vi "IV_Sweep_tool_Probe_Station_Resistance_measure_16_0202.vi"() -> ()   [LabVIEW 2013]
doc: "I. Description:\nThis example demonstrates how to continuously acquire and generate data at the same time, synchronized with one another.\n\nII. Instructions for Running:\n1. Select the physical channel to correspond to where your signal is input on the DAQ device. Also, select the corresponding channel for where your signal is being generated.\n2. Enter the minimum and maximum voltage ranges.\nNote: For better accuracy try to match the input range to the expected voltage level of the measured signal.\n3. Set the sample rate of the acquisition.\nNote: The rate should be at least twice as fast as the maximum frequency component of the signal being acquired. \n6. Select the Rate for the generation\n7. Select what type of signal to generate and the amplitude.\nNote: This example requires two DMA channels to run. If your hardware does not support two DMA channels, you need to set the Data Transfer Mechanism property for the Analog Output Task to use \"Interrupts\". The Data Transfer Mechanism property is located in the DAQmx Channel Property hierarchy at:\n\nDAQmx Channel Property Node>>Analog Output>>General Properties>>Advanced>>Data Transfer and Memory>>Data Transfer Mechanism\n\nRefer to your device documentation to determine how many DMA channels are supported for your hardware.\n\nIII. Block Diagram Steps:\n1. Create an analog input voltage channel. Also, create an analog output voltage channel.\n2. Set the rate for the sample clock. Additionally, define the sample mode to be continuous. Also, set the sample clock rate for the signal generation.\n2a. Call the Get Terminal Name with Device Prefix VI. This will take a Task and a terminal and create a properly formatted device + terminal name to use as the source of the Trigger.\n3. Define the parameters for a Digital Edge Start Trigger. Set the Analog output to trigger off the AI Start Trigger. This is an internal trigger signal.\n4. Use the Basic Function Generator VI to create the signal to be generated.\n5. Call the Start VI to arm the two functions. Make sure the analog output is armed before the analog input. This will ensure both will start at the same time.\n6. Read the waveform data in a loop until the user hits the stop button or an error occurs. The Is Task Done? VI is used to check for errors in the Analog Output Task.\n7. Call the Clear VI to Clear the Task\n8. Use the popup dialog box to display an error if any.\n\nIV. I/O Connections Overview:\nMake sure your signal input/output terminals match the Physical Channel I/O controls."
uses:
  <vilib>/Utility/error.llb/DialogType.ctl
  <vilib>/DAQmx/write.llb/DAQmx Write (Analog 2D DBL NChan NSamp).vi
  <vilib>/DAQmx/read.llb/DAQmx Read (Analog 1D DBL NChan 1Samp).vi
  <vilib>/DAQmx/write.llb/DAQmx Write (Analog DBL 1Chan 1Samp).vi
  <vilib>/DAQmx/read.llb/DAQmx Read (Analog DBL 1Chan 1Samp).vi
  <vilib>/Analysis/baseanly.llb/Mean (DBL).vi
  <vilib>/DAQmx/write.llb/DAQmx Write (Analog 1D DBL NChan 1Samp).vi
  <vilib>/DAQmx/create/channels.llb/DAQmx Create Channel (AO-Voltage-Basic).vi
  <vilib>/DAQmx/create/channels.llb/DAQmx Create Channel (AI-Voltage-Basic).vi
  <vilib>/DAQmx/configure/timing.llb/DAQmx Timing (Sample Clock).vi
  <vilib>/DAQmx/configure/trigger.llb/DAQmx Start Trigger (Digital Edge).vi
  <vilib>/DAQmx/miscellaneous.llb/DAQmx Fill In Error Info.vi
  <vilib>/Utility/file.llb/Write To Spreadsheet File (DBL).vi
  <vilib>/Utility/file.llb/Write To Spreadsheet File (string).vi
  pid/pid.llb/PID (DBL).vi
  pid/pid.llb/PID Output Rate Limiter (DBL).vi
  <vilib>/ptbypt/NI_PtbyPt.lvlib
  <resource>/objmgr/daqmx.rc
  <vilib>/Analysis/NI_AALBase.lvlib
  <vilib>/Analysis/NI_AALPro.lvlib
panel:
  in  "amplif":dbl=-0.01
  out "date/time string":string
  out "Bias Sweep 2":dbl[](graph)
  out "Array":dbl[](array[numeric])
  out "intercept":dbl
  out "Resistance":dbl
  out "RTD-IV":cluster{dbl[], dbl[]}(graph)
  in  "Bias Offset Correct":dbl
  out "Bias Sweep":dbl[](graph)
  out "element":dbl
  out "mean":dbl format="%.6f"
  out "size(s)":i32
  out "Numeric":i32
  in  "PID":bool=TRUE caption="Step Z"
  in  "Tab Control":enum32{"PID Controller", "Tapping Controls"}(tab)=enum."Tapping Controls"
  in  "Proportional Gain":dbl=0.0001
  in  "Integral Gain":dbl=1e-07
  in  "Differential Gain":dbl=1e-05
  in  "Setpoint":dbl=0.1
  in  "Piezo Delta rate":dbl=1000.0
  in  "Min Current":dbl=0.002
  in  "Max Current":dbl=10.2
  in  "Ramp Rate":dbl=20.0
  in  "Make Contact":i32=1200
  in  "Break Contact":i32=500
  in  "Step Length":i32=100
  in  "Step Max":dbl=0.3
  in  "Step Min":dbl=0.05
  out "Tapping Stop":bool
  out "Case":i32
  in  "Contact Cycles":i32
  in  "Tapping":bool caption="Step Z"
  out "x/y":dbl
  out "Waveform Chart":dbl(graph)
  in  "Analog Ouyput 1":dbl(slide) min=-10.0 max=10.0 step=0.001 scale=-10.0..10.0
  in  "Manual Z":bool caption="Step Z"
  in  "Sweep Amplitude":dbl=1.0
  in  "Stop Sweep":bool
  out "Connections 2":string="AI0=Current\nAI1=Bias\nAI2=dI/dV\nAI3=d2I/dV2\nAI4=X-Axis\nAI5=Z-Axis\n"
  out "Connections":string="AO0=Bias\nAO1=Z-axis\nAO2=X-Axis\nAO3=NA"
  out "Save Indicator":bool
  in  "Z-Direction":bool caption="Step Z"
  in  "Update Bias":bool
  in  "Save IV":bool
  in  "Save Decay":bool
  in  "Sweep Bias":bool
  in  "Step Z":bool
  in  "Comment":string="Molecule=TP4\nGain=10nA\nBias Gain=div/1\nSweep Freq.=0.0008Hz\nRef. Bias=4mV\nRef. Freq=2.977kHz\nGain LIA1=2mV\nTC LIA1=1s\nGain LIA2=5mV\nTC LIA2=1s\nLIA1=EGG\nLIA2=SRS\nEGG is driving(possible 5mV offset)"
  in  "Filenumber":i32
  in  "DATA Filename":string="Data_"
  in  "Data Directory":path=path "E:/Research/Data"
  out "Current Decay":cluster{dbl[], dbl[]}(graph)
  out "d2I/dV2":cluster{dbl[], dbl[]}(graph)
  out "dI/dV":cluster{dbl[], dbl[]}(graph)
  out "IV":cluster{dbl[], dbl[]}(graph)
  in  "# Samples":i32=2000
  in  "Frequency (Hz)":dbl=1.0
  out "Measurement 2":cluster{i32, dbl, dbl[]}(graph) caption="Measurement"
  out "Actual Update Generation Rate 2":dbl=5000.0 caption="Actual Update Generation Rate" format="%0.2f"
  in  "stop 3":bool
  in  "Bias":dbl=0.1 caption="Bias Start Point" step=0.1 format="%_3g"
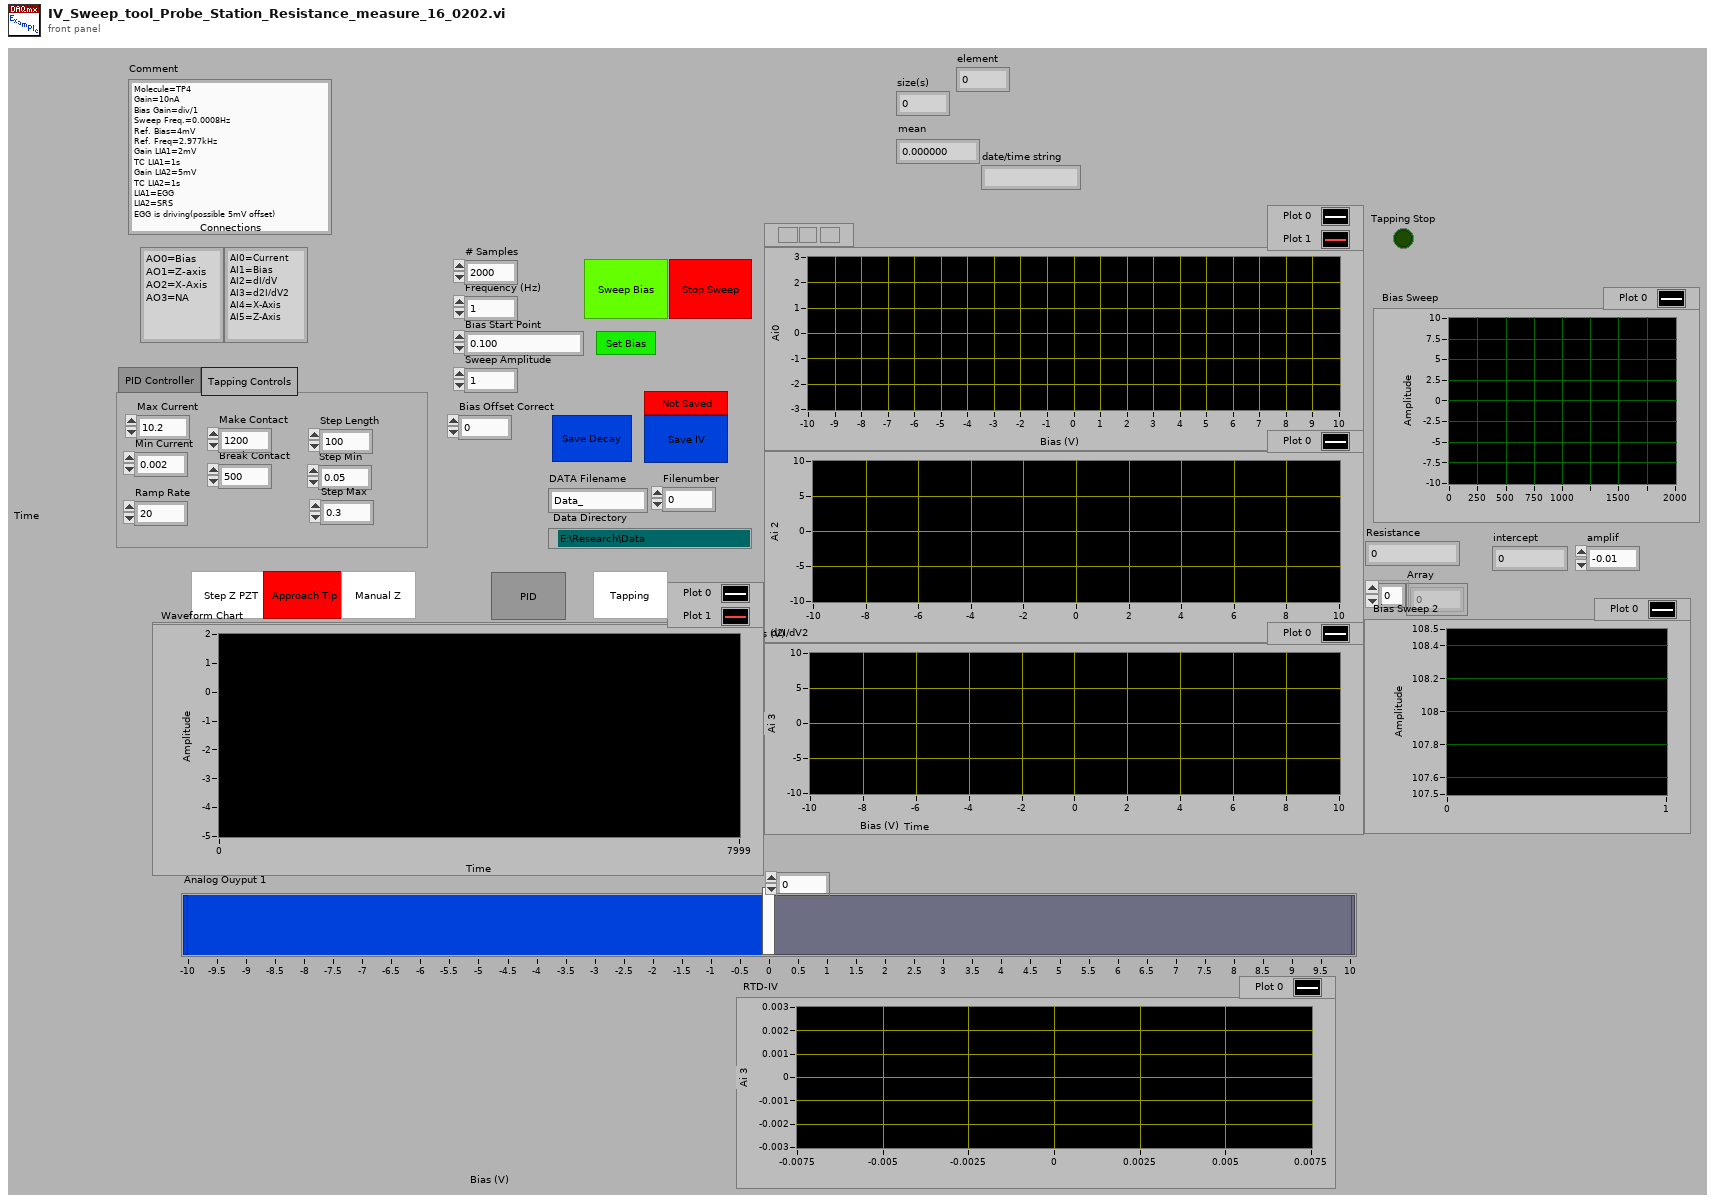
[diagram p1: front panel]
types:
  T1 = enum16{"open", "replace", "create", "open or create", "replace or create", "replace or create with confirmation"}
  T2 = typedef "DialogType.ctl" = u16
  T3 = cluster{"Proportional Gain":dbl, "Integral Gain ":dbl, "Differential Gain":dbl}
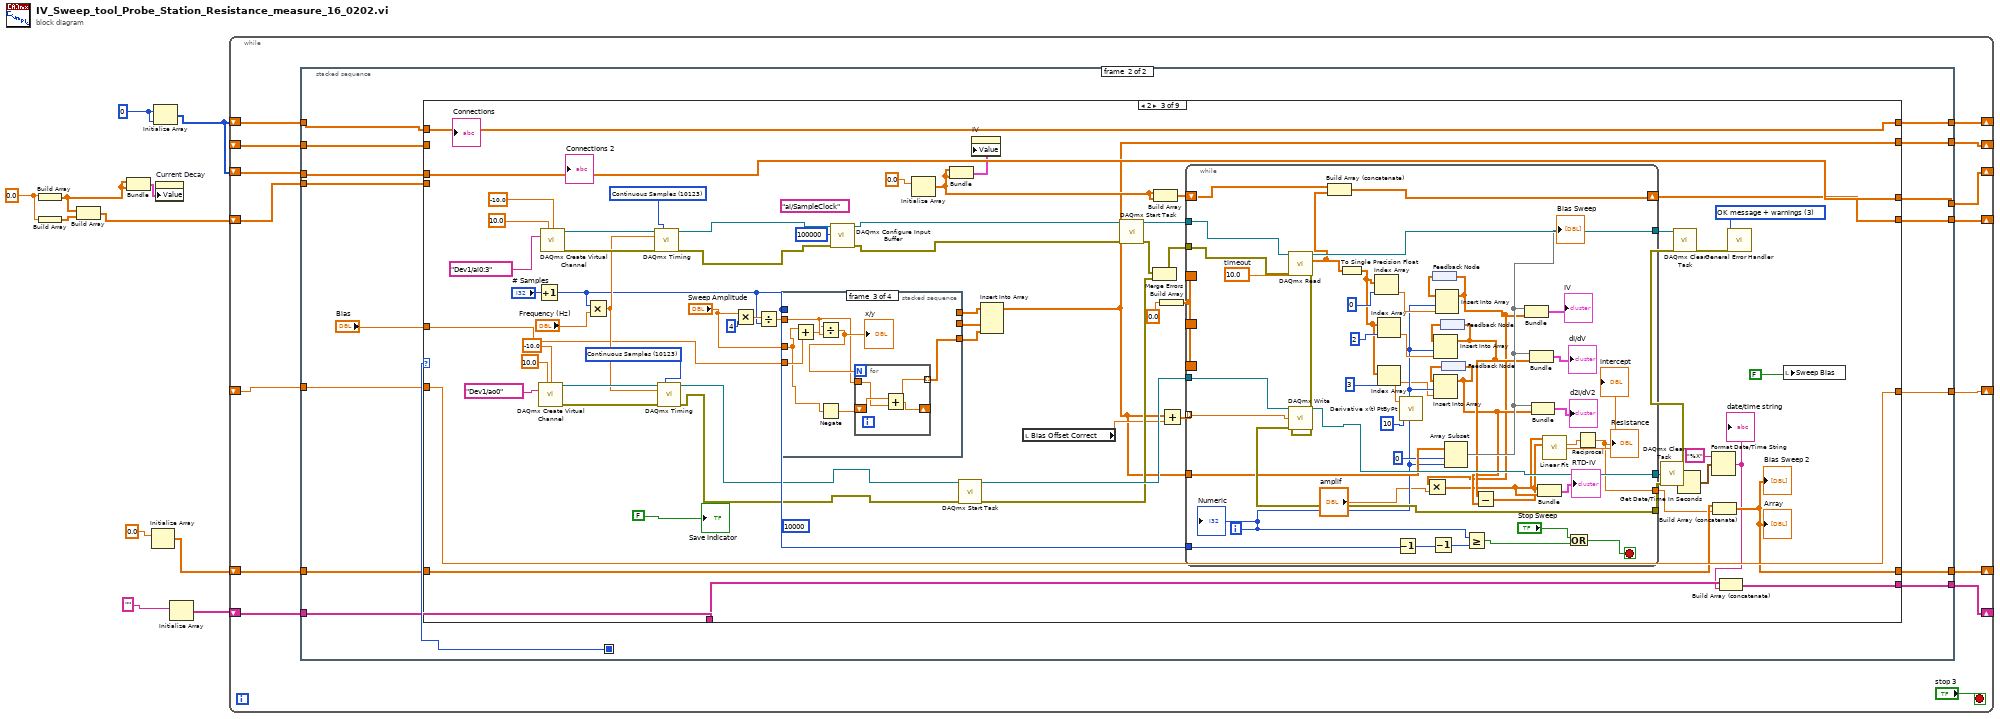
[diagram p0: block diagram]
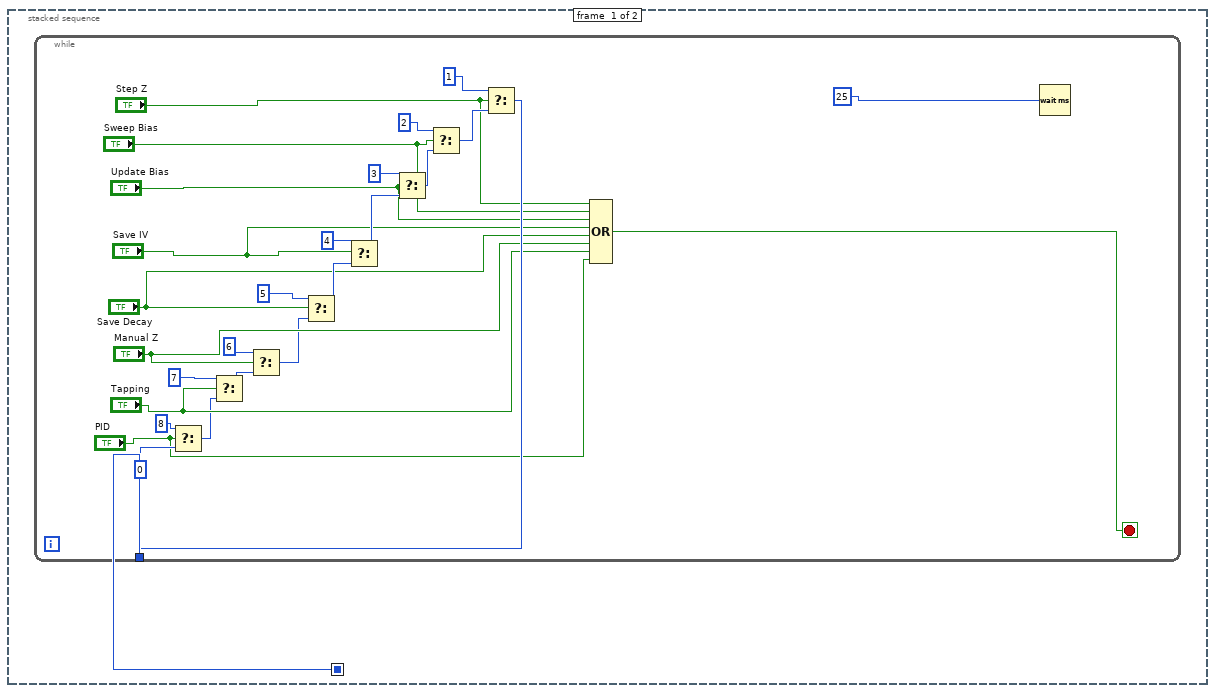
[diagram p2: hidden frame]
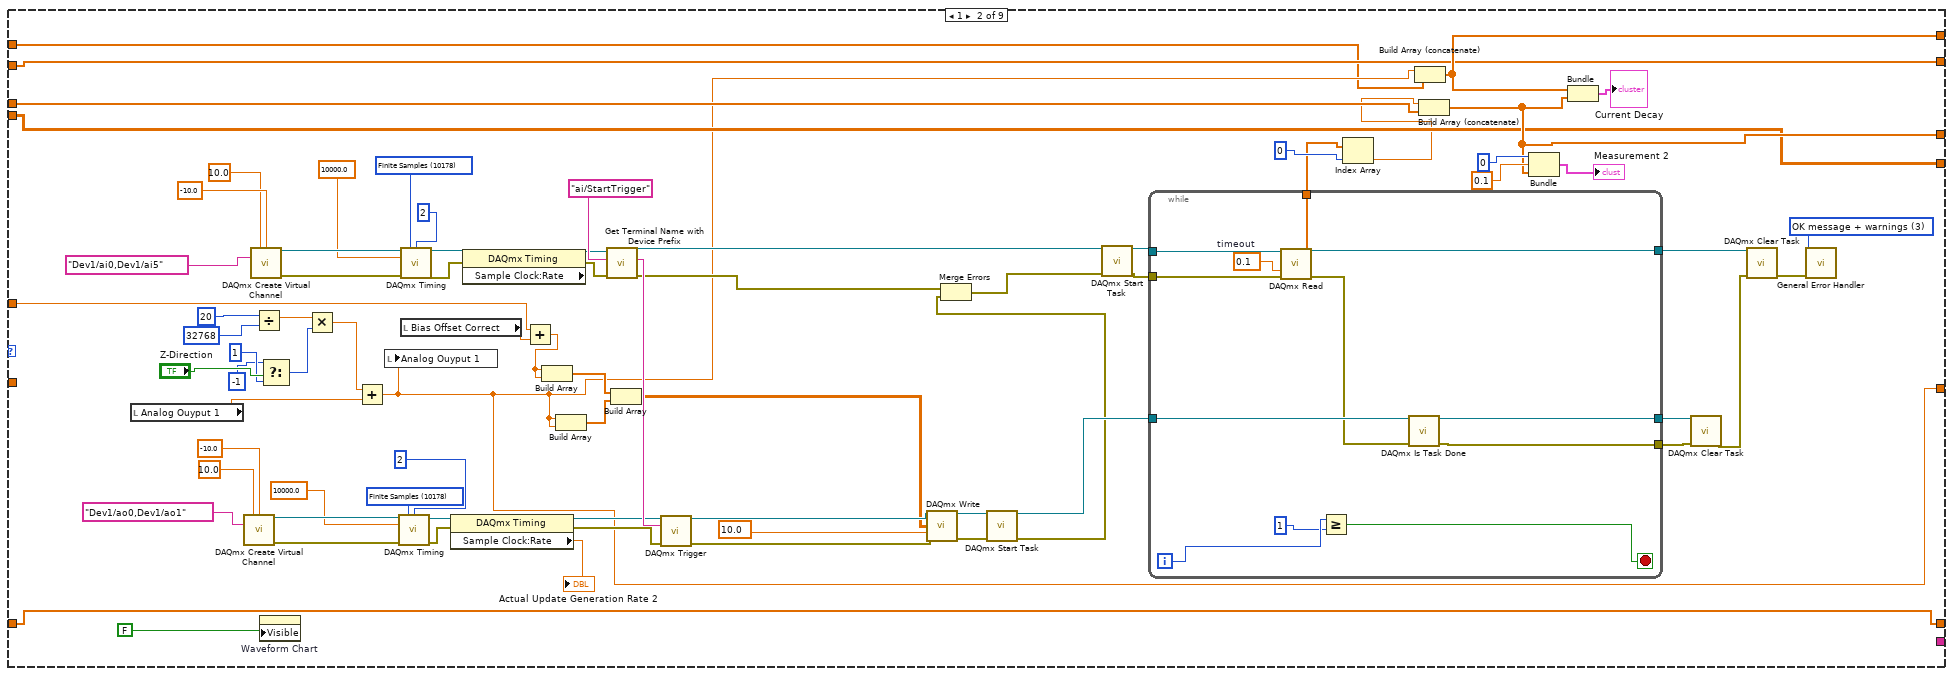
[diagram p4: hidden frame]
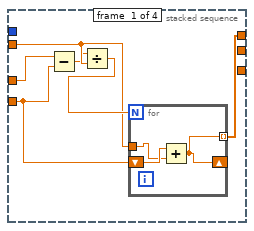
[diagram p5: hidden frame]
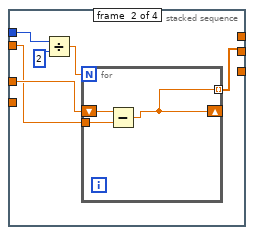
[diagram p6: hidden frame]
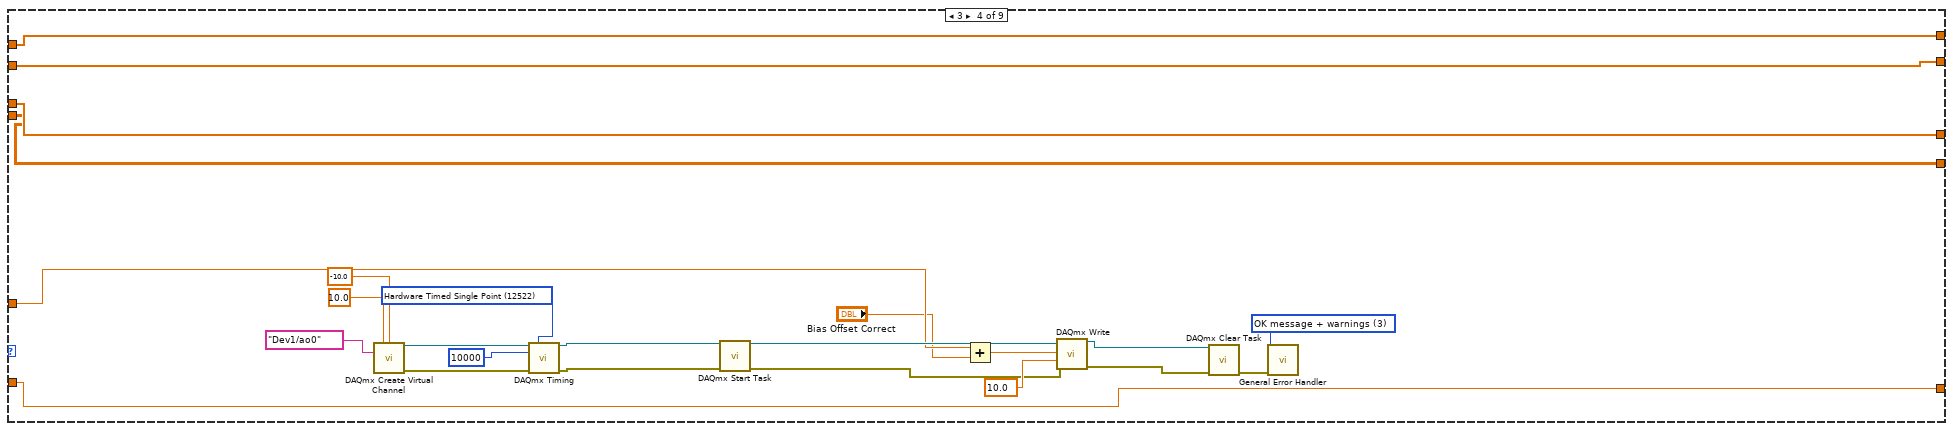
[diagram p8: hidden frame]
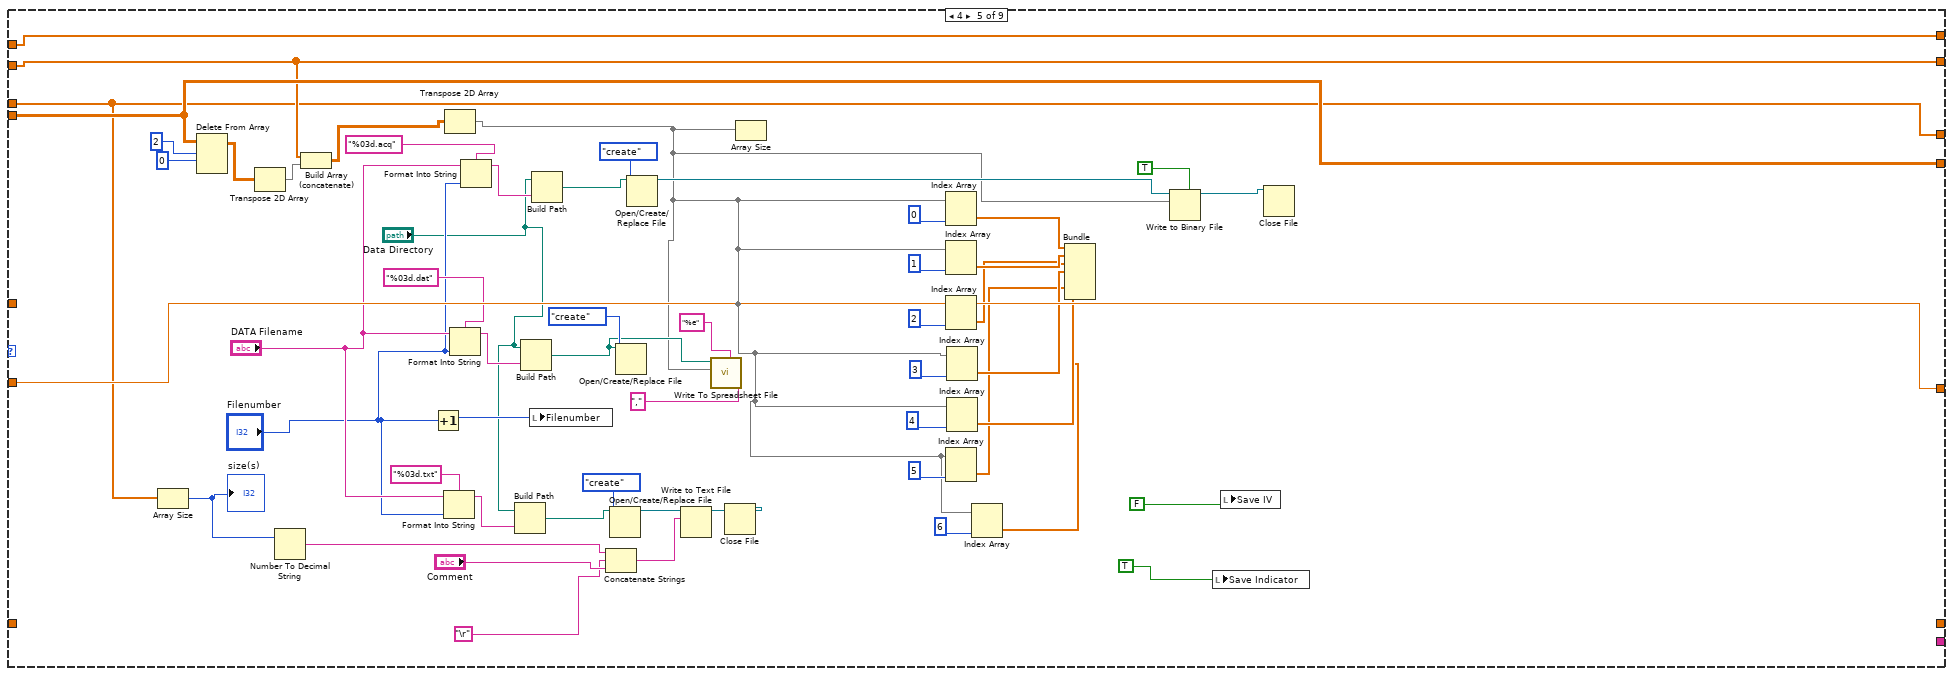
[diagram p9: hidden frame]
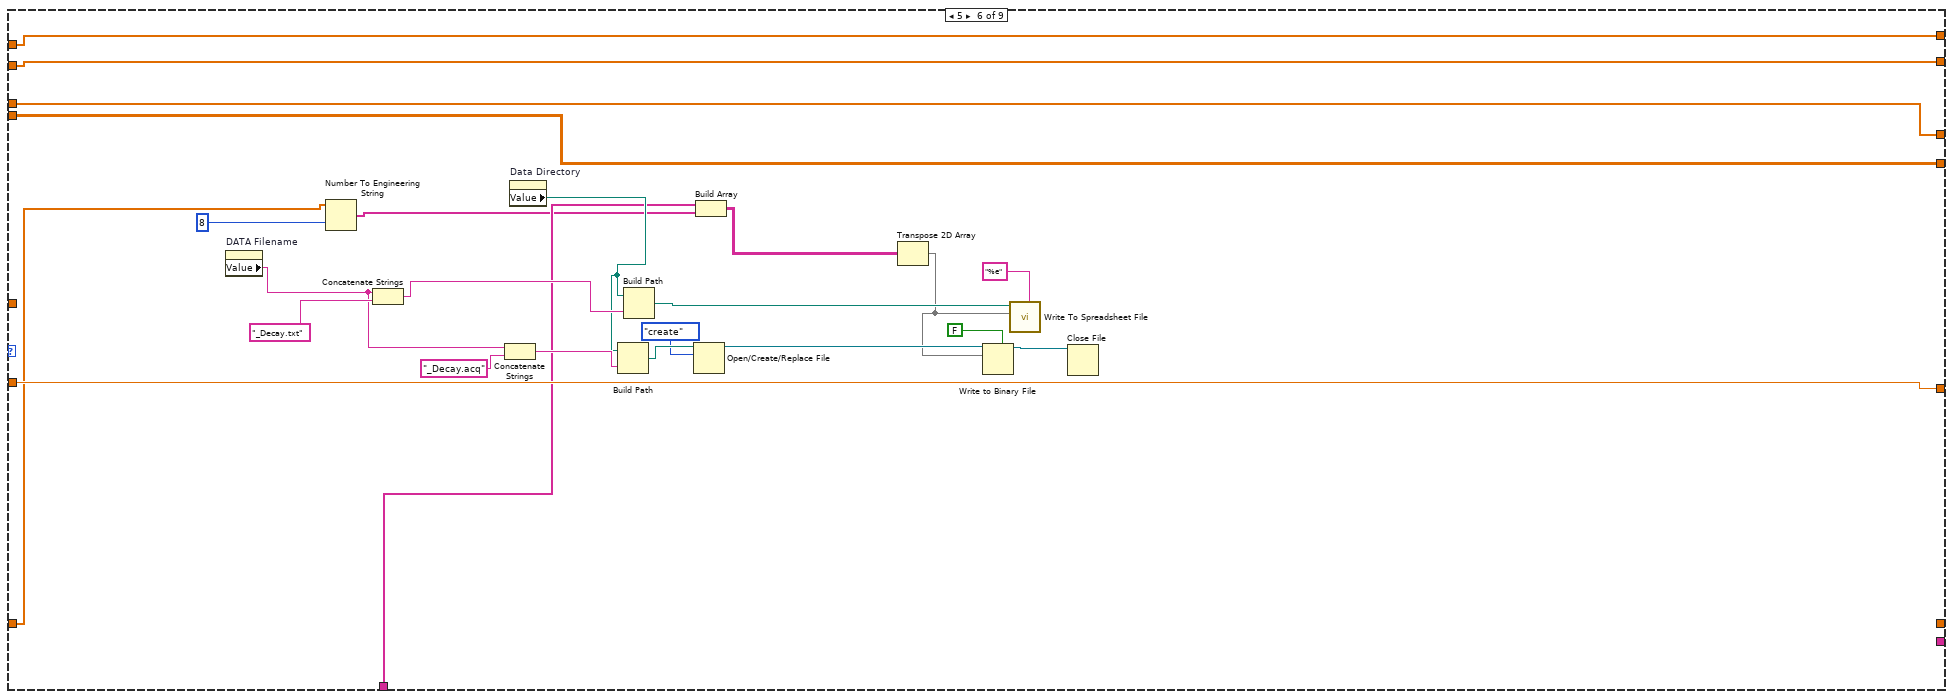
[diagram p10: hidden frame]
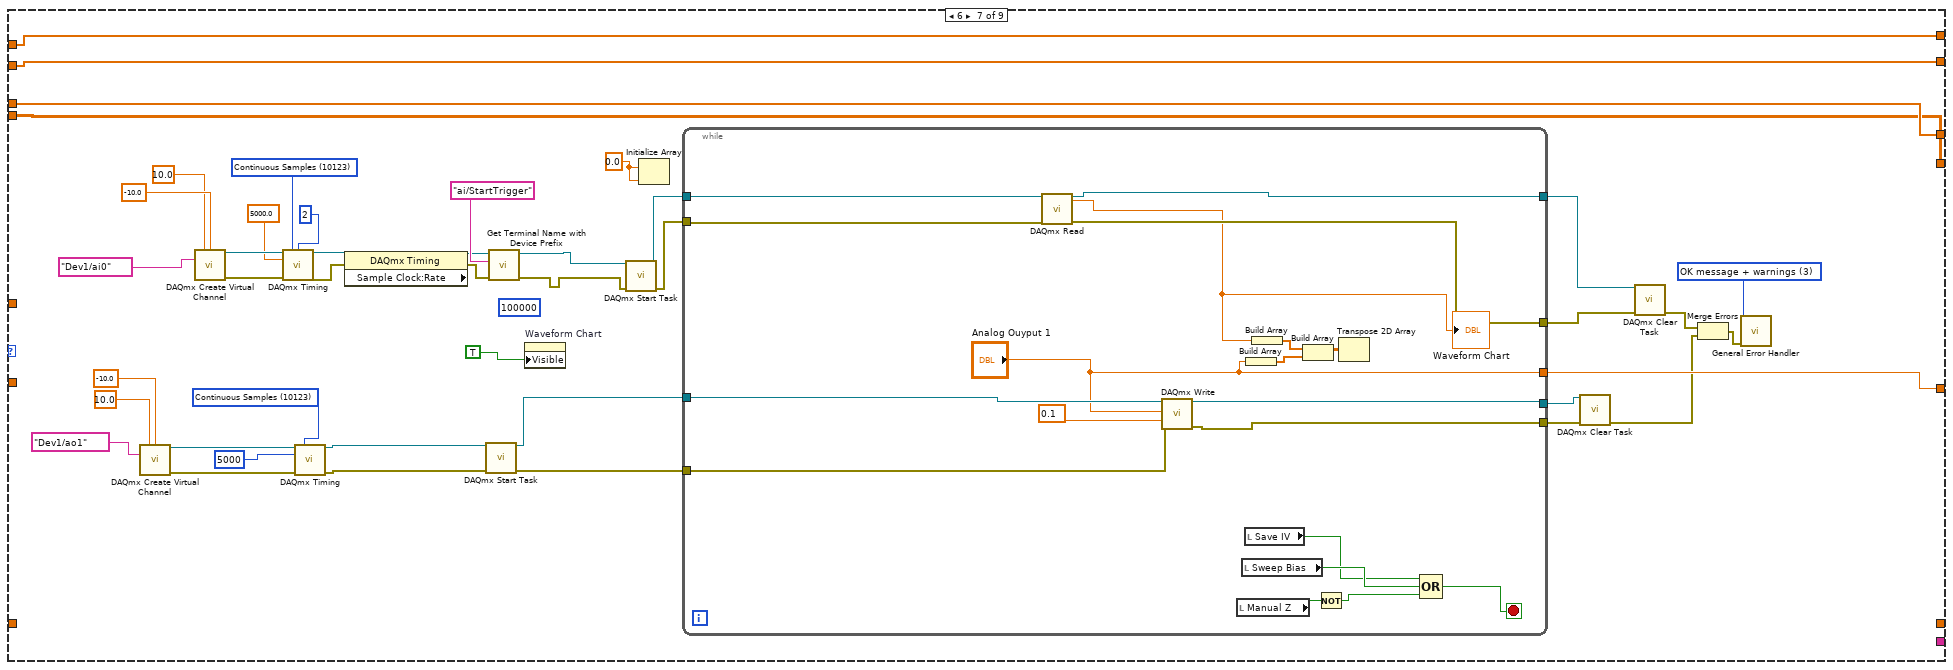
[diagram p11: hidden frame]
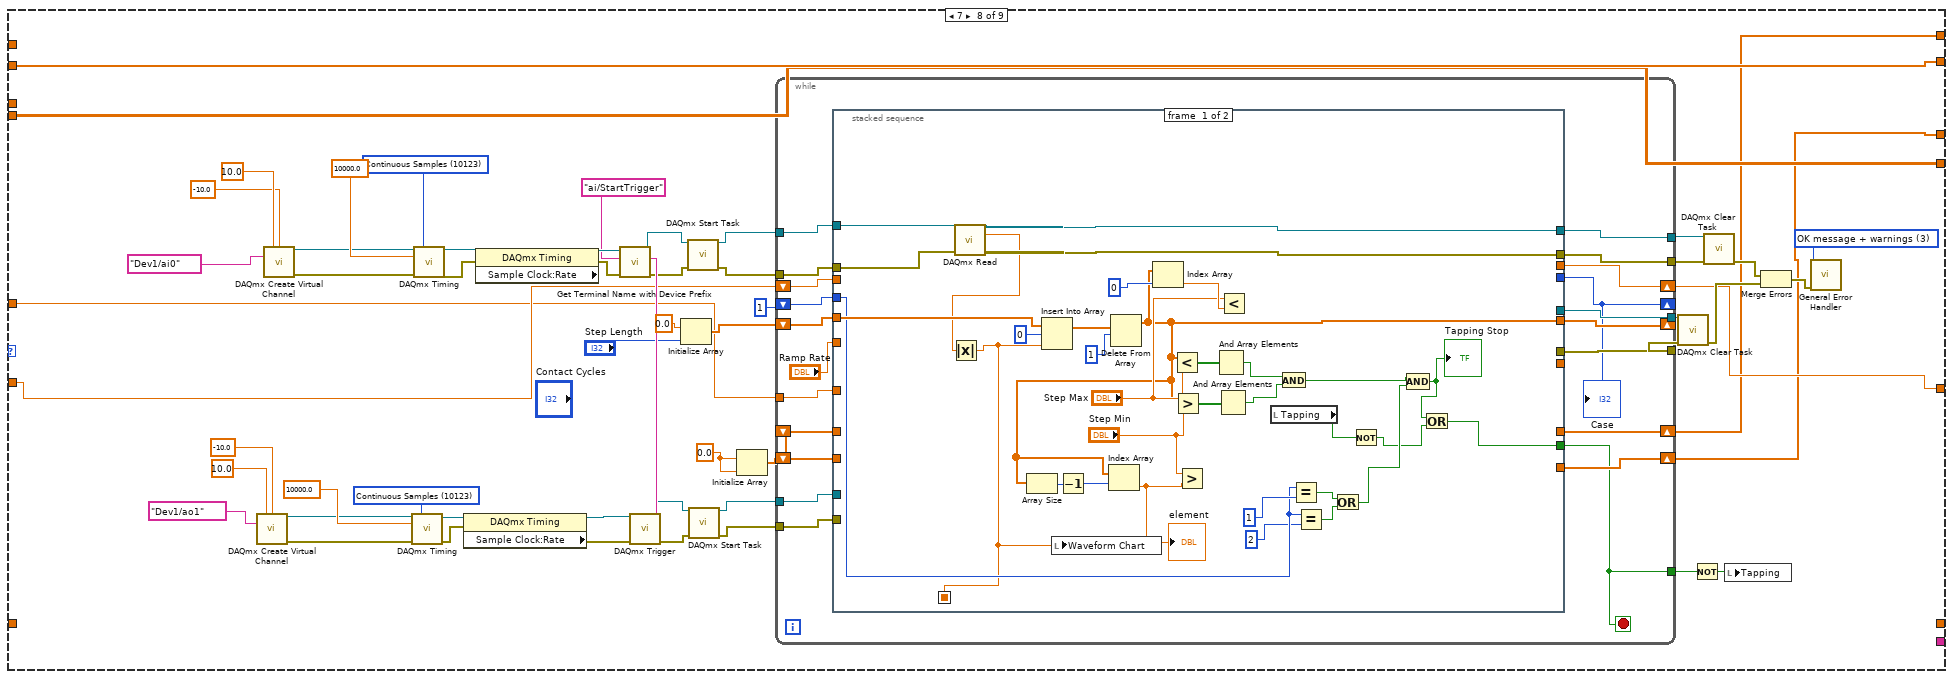
[diagram p12: hidden frame]
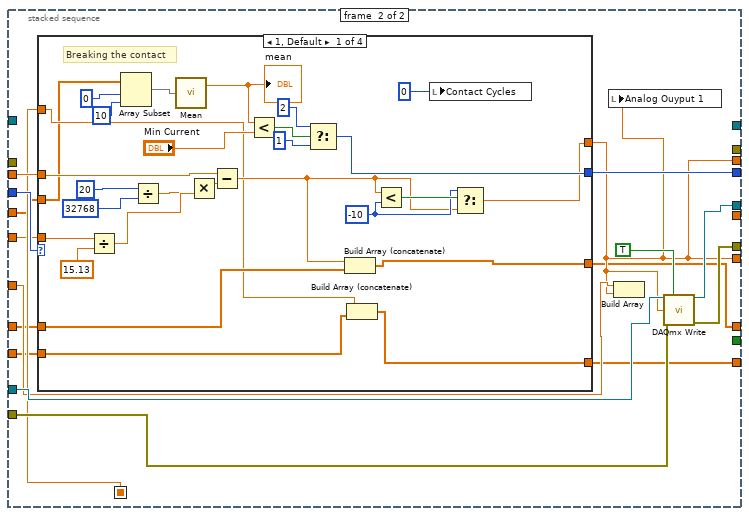
[diagram p13: hidden frame]
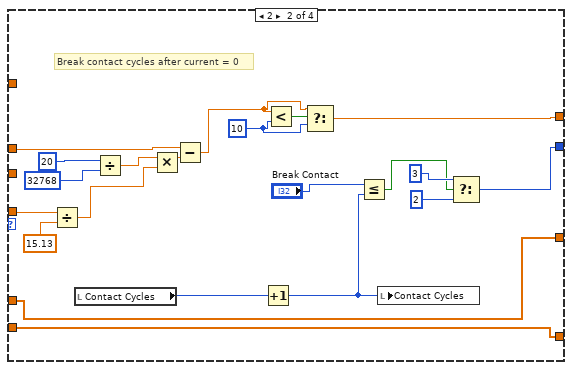
[diagram p14: hidden frame]
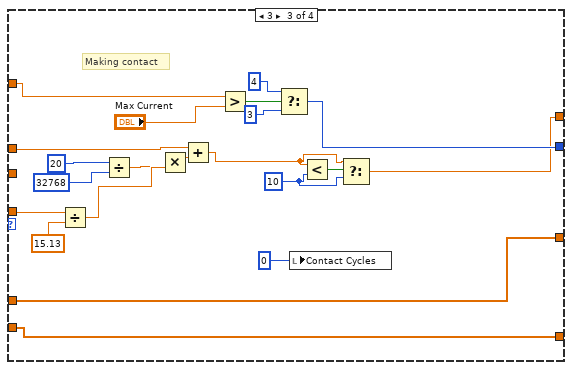
[diagram p15: hidden frame]
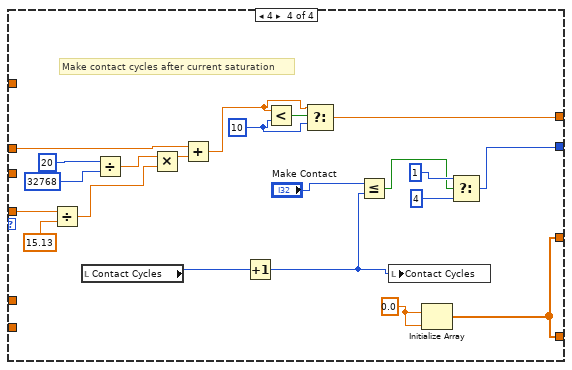
[diagram p16: hidden frame]
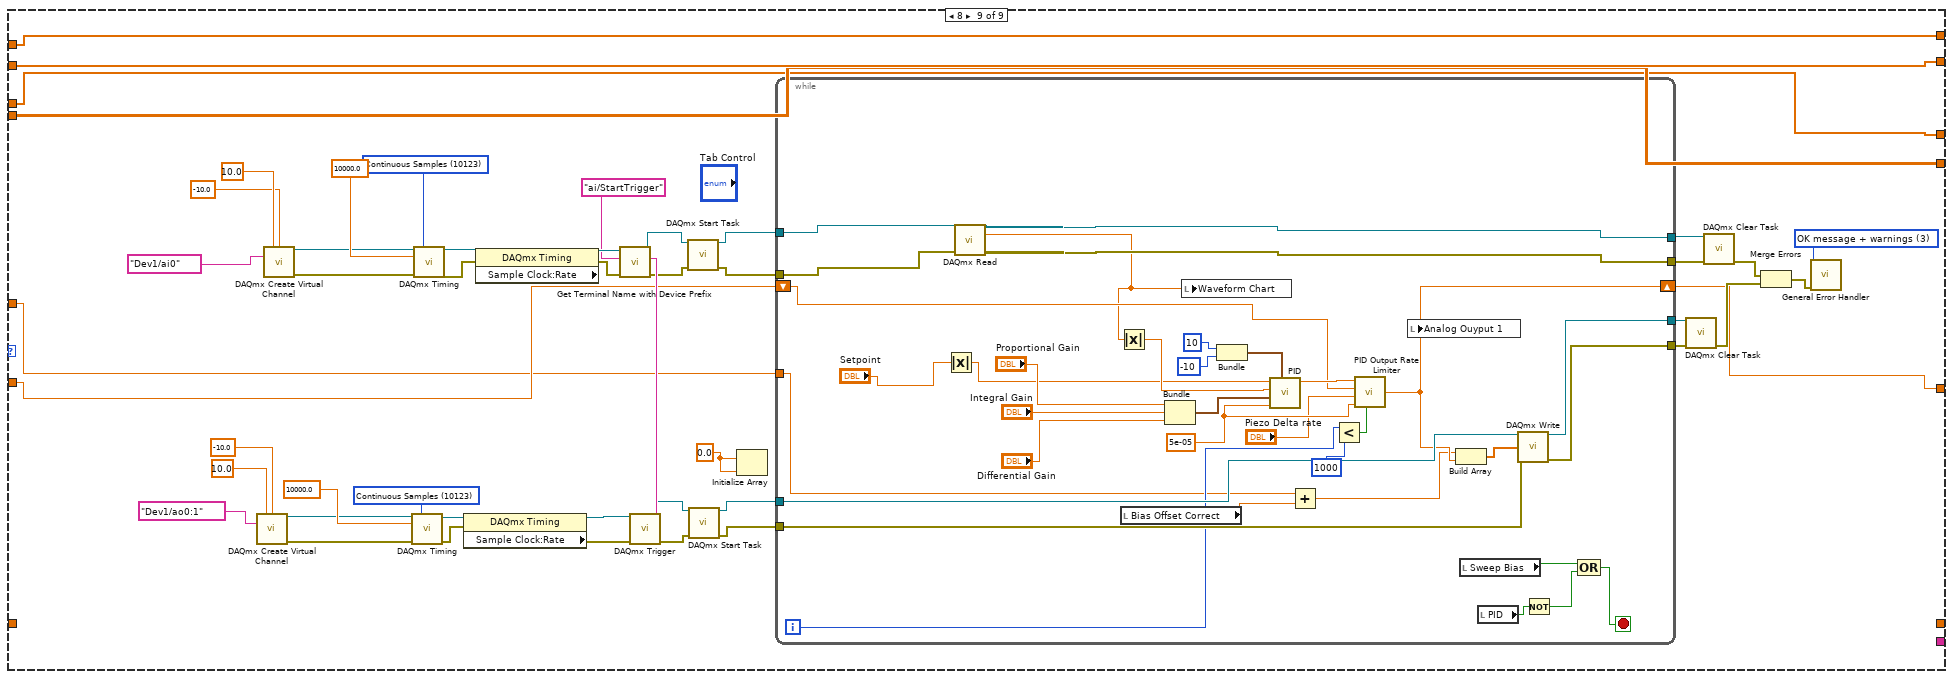
[diagram p17: hidden frame]
diagram:
  w6 = 0
  w11 = 0.0
  n1 = Build Array(w11) -> (w8:dbl[])
  n2 = Build Array(w11) -> (w10:dbl[])
  n3 = Build Array(w8, w10) -> (w9:dbl[][])
  n4 = Bundle(w8, w8) -> (w7:cluster{dbl[], dbl[]})  [unwired: 1 in]
  n5 = Initialize Array(0.0) -> (w3:dbl[])  [unwired: 1 in]
  n6 = Initialize Array(w6, w6) -> (w5:i32[])
  n7 = property on="Current Decay" class="XYGraph (strict)"("Value"=w7) -> ()  [unwired: 2 in, 2 out]
  n8 = Initialize Array("") -> (w1:string[])  [unwired: 1 in]
  n9 = while {
    shift-right: [w24] -> _
    shift-left: w5 -> [w25]
    shift-right: [w22] -> _
    shift-left: w5 -> [w23]
    shift-right: [w20] -> _
    shift-left: _ -> [w21]
    shift-right: [w18] -> _
    shift-left: w9 -> [w19]
    shift-right: [w16] -> _
    shift-left: _ -> [w17]
    shift-right: [w15] -> _
    shift-left: w3 -> [w14]
    shift-right: [w12] -> _
    shift-left: w1 -> [w13]
    stop <- "stop 3" stop-if-true
    n10 = stacked-sequence {
      seq-local: [w27 _] -> [_ w70]
      tunnel: w25 -> [_ w69]
      tunnel: [_ w68] -> w24
      tunnel: w23 -> [_ w66]
      tunnel: [_ w65] -> w22
      tunnel: w21 -> [_ w64]
      tunnel: [_ w59] -> w20
      tunnel: w19 -> [_ w63]
      tunnel: [_ w62] -> w18
      tunnel: w17 -> [_ w61]
      tunnel: [_ w60] -> w16
      tunnel: w14 -> [_ w58]
      tunnel: [_ w57] -> w15
      tunnel: w13 -> [_ w56]
      tunnel: [_ w55] -> w12
      frame #0 {
        n11 = while {
          tunnel: [w45] -> w27
          stop <- w44 stop-if-true
          n12 = Select(t=8, s="PID", f=0) -> (s? t:f=w31:i32)
          n13 = Select(t=7, s="Tapping", f=w31) -> (s? t:f=w33:i32)
          n14 = Select(t=6, s="Manual Z", f=w33) -> (s? t:f=w34:i32)
          n15 = Select(t=5, s="Save Decay", f=w34) -> (s? t:f=w50:i32)
          n16 = Select(t=4, s="Save IV", f=w50) -> (s? t:f=w49:i32)
          n17 = Select(t=3, s="Update Bias", f=w49) -> (s? t:f=w47:i32)
          n18 = Select(t=2, s="Sweep Bias", f=w47) -> (s? t:f=w54:i32)
          n19 = Select(t=1, s="Step Z", f=w54) -> (s? t:f=w45:i32)
          n20 = Compound Arithmetic op=OR("Step Z", "Sweep Bias", "Update Bias", "Save IV", "Save Decay", "Manual Z", "Tapping", "PID") -> (w44:bool)
          n21 = Wait (ms)(milliseconds to wait=25) -> ()  [unwired: 1 out]
        }
      }
      frame #1 {
        n22 = case shown="2" w70 {
          tunnel: w69 -> [w77 w85 w214 w312 w332 w388 w448 _ w688]
          tunnel: [w77 w98 w214 w312 w332 w388 w448 w474 w688] -> w68
          tunnel: "Bias" -> [_ w81 w199 w306 _ _ _ w480 w687]
          tunnel: w66 -> [w76 w82 w211 w313 w379 w404 w450 _ w689]
          tunnel: [w76 w99 w211 w313 w379 w404 w450 w475 w689] -> w65
          tunnel: w64 -> [w75 _ w210 w311 w378 w405 _ w481 w696]
          tunnel: [w75 w83 w210 w311 w378 w405 w419 w476 w693] -> w59
          tunnel: w63 -> [w74 w96 _ w309 w358 w406 w447 w478 w694]
          tunnel: [w74 w96 w191 w309 w358 w406 w447 w478 w694] -> w62
          tunnel: [w73 w91 w174 w308 w356 w389 w449 w479 w695] -> w60
          tunnel: w61 -> [w73 w91 _ w308 w356 w389 w449 w479 w695]
          tunnel: w58 -> [w72 w78 w173 _ _ w386 _ _ _]
          tunnel: [w72 w78 w171 _ _ _ _ _ _] -> w57
          tunnel: w56 -> [w71 _ w170 _ _ w387 _ _ _]
          tunnel: [w71 _ w169 _ _ _ _ _ _] -> w55
          frame 0, Default {
          }
          frame 1 {
            w133 = T2 3 items=["no dialog", "OK message", "continue or stop message", "OK message + warnings", "continue/stop + warnings"] ("type of dialog (OK msg:1)")
            w145 = 10178 items=["Finite Samples"=10178, "Continuous Samples"=10123] ("sample mode")
            w150 = 10178 items=["Finite Samples"=10178, "Continuous Samples"=10123] ("sample mode")
            n23 = local read "Analog Ouyput 1"() -> (w86:dbl)
            n24 = call-poly <vilib>:"DAQmx Create Virtual Channel.vi"("maximum value"=10.0 ("maximum value 2"), "minimum value"=-10.0 ("minimum value 2"), "physical channels"=tag "Dev1/ao0,Dev1/ao1" ("physical channels 2")) -> ("task out"=w144:refnum<k21>, "error out"=w143:errorcluster)  [unwired: 11 in]
            n25 = call-poly <vilib>:"DAQmx Create Virtual Channel.vi"("maximum value"=10.0 ("Maximum Value 2"), "minimum value"=-10.0 ("Minimum Value 2"), "physical channels"=tag "Dev1/ai0,Dev1/ai5" ("Physical Channel 2")) -> ("task out"=w148:refnum<k21>, "error out"=w149:errorcluster)  [unwired: 11 in]
            n26 = Divide(x=20, y=32768) -> (x/y=w95:dbl)
            n27 = property on="Waveform Chart" class="WFChart (strict)"("Visible"=FALSE) -> ()  [unwired: 2 in, 2 out]
            n28 = Select(t=-1 ("f"), s="Z-Direction", f=1) -> (s? t:f=w93:i32)
            n29 = Multiply(x=w95, y=w93) -> (x*y=w94:dbl)
            n30 = Add(x=w94, y=w86) -> (x+y=w83:dbl)
            n31 = local write "Analog Ouyput 1"(w83) -> ()
            n32 = call-poly <vilib>:"DAQmx Timing.vi"("task/channels in"=w144, "sample mode"=w145, "samples per channel"=2, "rate"=10000.0 ("rate 2"), "error in"=w143) -> ("task out"=w128:refnum<k21>, "error out"=w127:errorcluster)  [unwired: 9 in]
            n33 = call-poly <vilib>:"DAQmx Timing.vi"("task/channels in"=w148, "sample mode"=w150, "samples per channel"=2, "rate"=10000.0 ("Rate 2"), "error in"=w149) -> ("task out"=w122:refnum<k21>, "error out"=w121:errorcluster)  [unwired: 9 in]
            n34 = local read "Bias Offset Correct"() -> (w80:dbl)
            n35 = property class="DAQmx Timing"(reference=w128, error in=w127) -> (reference out=w129:refnum<k21>, error out=w126:errorcluster, "Sample Clock:Rate"=→"Actual Update Generation Rate 2":dbl)
            n36 = property class="DAQmx Timing" props=["Sample Clock:Rate"](reference=w122, error in=w121) -> (reference out=w120:refnum<k21>, error out=w119:errorcluster)  [unwired: 1 out]
            n37 = Add(x=w81, y=w80) -> (x+y=w79:dbl)
            n38 = Build Array(w79, w79) -> (w106:dbl[])
            n39 = Build Array(w83, w83) -> (w105:dbl[])
            n40 = call "Get Terminal Name with Device Prefix.vi"("error in (no error)"=w119, "Local Terminal Name"="ai/StartTrigger" ("terminal"), "task/channels in"=w120) -> ("error out"=w125:errorcluster, "Terminal Name with Device Prefix"=w130:tag, "task out"=w110:refnum<k21>)  [unwired: 6 in]
            n41 = Build Array(w106, w105) -> (w104:dbl[][])
            n42 = call-poly <vilib>:"DAQmx Trigger.vi"("task/channels in"=w129, "source"=w130, "error in"=w126) -> ("task out"=w135:refnum<k21>, "error out"=w136:errorcluster)  [unwired: 11 in]
            n43 = call-poly <vilib>:"DAQmx Write.vi"("task/channels in"=w135, "data"=w104, "timeout"=10.0 ("Wirite Timeout"), "error in"=w136) -> ("task out"=w138:refnum<k21>, "error out"=w137:errorcluster)  [unwired: 9 in, 1 out]
            n44 = call <vilib>:"DAQmx Start Task.vi"("task/channels in"=w138, "error in"=w137) -> ("task out"=w142:refnum<k21>, "error out"=w124:errorcluster)  [unwired: 12 in]
            n45 = Merge Errors(w125, w124) -> (w112:errorcluster)
            n46 = call <vilib>:"DAQmx Start Task.vi"("task/channels in"=w110, "error in"=w112) -> ("task out"=w109:refnum<k21>, "error out"=w111:errorcluster)  [unwired: 12 in]
            n47 = while {
              tunnel: [w165] -> w151
              tunnel: w142 -> [w164]
              tunnel: [w163] -> w141
              tunnel: w109 -> [w154]
              tunnel: [w162] -> w118
              tunnel: [w159] -> w102
              tunnel: w111 -> [w155]
              i -> [w158]
              stop <- w156 stop-if-true
              w161 = 0.1  # timeout
              n48 = call-poly <vilib>:"DAQmx Read.vi"("task/channels in"=w154, "timeout"=w161, "error in"=w155) -> ("task out"=w165:refnum<k21>, "data"=w159:dbl[], "error out"=w160:errorcluster)  [unwired: 10 in]
              n49 = Greater Or Equal?(x=w158, y=1) -> (x >= y?=w156:bool)
              n50 = call <vilib>:"DAQmx Is Task Done.vi"("task/channels in"=w164, "error in"=w160) -> ("task out"=w163:refnum<k21>, "error out"=w162:errorcluster)  [unwired: 11 in, 1 out]
            }
            n51 = Index Array(array=w102, index=0) -> (element=w84:dbl)
            n52 = Build Array (concatenate)(w83, w82) -> (w99:dbl[])
            n53 = Build Array (concatenate)(w84, w85) -> (w98:dbl[])
            n54 = Bundle(0, 0.1, w98) -> (→"Measurement 2":cluster{i32, dbl, dbl[]})  [unwired: 1 in]
            n55 = Bundle(w99, w98) -> (→"Current Decay":cluster{dbl[], dbl[]})  [unwired: 1 in]
            n56 = call <vilib>:"DAQmx Clear Task.vi"("task in"=w141, "error in"=w118) -> ("error out"=w117:errorcluster)  [unwired: 13 in]
            n57 = call <vilib>:"DAQmx Clear Task.vi"("task in"=w151, "error in"=w117) -> ("error out"=w116:errorcluster)  [unwired: 13 in]
            n58 = call <vilib>:"General Error Handler.vi"("type of dialog (OK msg:1)"=w133, "error in (no error)"=w116) -> ()  [unwired: 9 in, 5 out]
          }
          frame 2 {
            (unwired) 10000
            w208 = 10123 items=["Finite Samples"=10178, "Continuous Samples"=10123, "Hardware Timed Single Point"=12522] ("sample mode")
            w209 = 10123 items=["Finite Samples"=10178, "Continuous Samples"=10123, "Hardware Timed Single Point"=12522] ("sample mode")
            (unwired) "ai/SampleClock" ("terminal")
            w219 = T2 3 items=["no dialog", "OK message", "continue or stop message", "OK message + warnings", "continue/stop + warnings"] ("type of dialog (OK msg:1)")
            n59 = Increment(x="# Samples") -> (x+1=w189:i32)
            n60 = call-poly <vilib>:"DAQmx Create Virtual Channel.vi"("maximum value"=10.0, "minimum value"=-10.0, "physical channels"=tag "Dev1/ao0") -> ("task out"=w222:refnum<k21>, "error out"=w221:errorcluster)  [unwired: 11 in]
            n61 = call-poly <vilib>:"DAQmx Create Virtual Channel.vi"("maximum value"=10.0 ("Maximum Value"), "minimum value"=-10.0 ("Minimum Value"), "physical channels"=tag "Dev1/ai0:3" ("Physical Channel")) -> ("task out"=w226:refnum<k21>, "error out"=w227:errorcluster)  [unwired: 11 in]
            n62 = Multiply(x=w189, y="Frequency (Hz)") -> (x*y=w213:dbl)
            n63 = call-poly <vilib>:"DAQmx Timing.vi"("task/channels in"=w226, "sample mode"=w208, "rate"=w213, "error in"=w227) -> ("task out"=w183:refnum<k21>, "error out"=w181:errorcluster)  [unwired: 10 in]
            n64 = call-poly <vilib>:"DAQmx Timing.vi"("task/channels in"=w222, "sample mode"=w209, "rate"=w213, "error in"=w221) -> ("task out"=w178:refnum<k21>, "error out"=w177:errorcluster)  [unwired: 10 in]
            n65 = Multiply(x="Sweep Amplitude", y=4) -> (x*y=w197:dbl)
            n66 = Divide(x=w197, y=w189) -> (x/y=w196:dbl)
            n67 = stacked-sequence {
              tunnel: "Sweep Amplitude" -> [w282 w288 w296 _]
              tunnel: w199 -> [w280 _ w300 _]
              tunnel: w196 -> [w278 w287 w298 _]
              tunnel: [w279 _ _ _] -> w195
              tunnel: w189 -> [_ w291 _ _]
              tunnel: [_ w286 _ _] -> w194
              tunnel: [_ _ w299 _] -> w193
              frame #0 {
                n68 = Subtract(x=w282, y=w280) -> (x-y=w277:dbl)
                n69 = Divide(x=w277, y=w278) -> (x/y=w281:dbl)
                n70 = for {
                  N: w281 -> [_]
                  tunnel: w278 -> [w284]
                  shift-right: [w283] -> _
                  shift-left: w280 -> [w285]
                  tunnel: [w283] -> w279 mode=indexing
                  n71 = Add(x=w285, y=w284) -> (x+y=w283:dbl)
                }
              }
              frame #1 {
                n72 = Divide(x=w291, y=2) -> (x/y=w289:dbl)
                n73 = for {
                  N: w289 -> [_]
                  tunnel: w287 -> [w293]
                  shift-right: [w292] -> _
                  shift-left: w288 -> [w294]
                  tunnel: [w292] -> w286 mode=indexing
                  n74 = Subtract(x=w294, y=w293) -> (x-y=w292:dbl)
                }
              }
              frame #2 {
                n75 = Add(x=w296, y=w300) -> (x+y=w297:dbl)
                n76 = Divide(x=w297, y=w298) -> (x/y=w301:dbl)
                "x/y" <- w301
                n77 = Negate(x=w296) -> (-x=w295:dbl)
                n78 = for {
                  N: w301 -> [_]
                  tunnel: w298 -> [w303]
                  shift-right: [w302] -> _
                  shift-left: w295 -> [w304]
                  tunnel: [w302] -> w299 mode=indexing
                  n79 = Add(x=w304, y=w303) -> (x+y=w302:dbl)
                }
              }
              frame #3 {
              }
            }
            n80 = call <vilib>:"DAQmx Configure Input Buffer.vi"("task/channels in"=w183, "buffer size (in samples per channel)"=100000, "error in"=w181) -> ("task out"=w182:refnum<k21>, "error out"=w180:errorcluster)  [unwired: 11 in]
            n81 = Initialize Array(0.0) -> (w188:dbl[])  [unwired: 1 in]
            n82 = Bundle(w188, w188) -> (w187:cluster{dbl[], dbl[]})  [unwired: 1 in]
            n83 = call <vilib>:"DAQmx Start Task.vi"("task/channels in"=w178, "error in"=w177) -> ("task out"=w207:refnum<k21>, "error out"=w203:errorcluster)  [unwired: 12 in]
            n84 = property on="IV" class="XYGraph (strict)"("Value"=w187) -> ()  [unwired: 2 in, 2 out]
            n85 = Insert Into Array(array=w195, new element #1=w194, new element #2=w193) -> (w174:dbl[])  [unwired: 1 in]
            n86 = local read "Bias Offset Correct"() -> (w175:dbl)
            n87 = call <vilib>:"DAQmx Start Task.vi"("task/channels in"=w182, "error in"=w180) -> ("task out"=w205:refnum<k21>, "error out"=w204:errorcluster)  [unwired: 12 in]
            n88 = Merge Errors(w204, w203) -> (w206:errorcluster)
            n89 = Build Array(w188, w188) -> (w190:dbl[][])
            n90 = Build Array(0.0) -> (w185:dbl[])
            n91 = Add(x=w174, y=w175) -> (x+y=w176:dbl[])
            n92 = while {
              tunnel: [w268] -> w228
              tunnel: [w271] -> w220
              tunnel: [w270] -> w217
              tunnel: w189 -> [w246]
              tunnel: w176 -> [w251] mode=indexing
              tunnel: w207 -> [w273]
              tunnel: w205 -> [w276]
              tunnel: w206 -> [w275]
              shift-right: [w252] -> w191
              shift-left: w190 -> [w269]
              tunnel: w174 -> [w266]
              border: w185 -> [_]
              border: w185 -> [_]
              border: w185 -> [_]
              tunnel: [w232] -> w172
              i -> [w247]
              stop <- w248 stop-if-true
              w272 = 10.0  # timeout
              n93 = call-poly <vilib>:"DAQmx Read.vi"("task/channels in"=w276, "timeout"=w272, "error in"=w275) -> ("task out"=w268:refnum<k21>, "data"=w254:dbl[], "error out"=w274:errorcluster)  [unwired: 10 in]
              n94 = call-poly <vilib>:"DAQmx Write.vi"("task/channels in"=w273, "data"=w251, "error in"=w274) -> ("task out"=w271:refnum<k21>, "error out"=w270:errorcluster)  [unwired: 10 in, 1 out]
              n95 = Build Array (concatenate)(w269, w254) -> (w252:dbl[][])
              n96 = To Single Precision Float(number=w254) -> (single precision float=w253:sgl[])
              n97 = Index Array(array=w253, index=0) -> (element=w264:sgl)
              n98 = Index Array(array=w253, index=2) -> (element=w260:sgl)
              n99 = Index Array(array=w253, index=3) -> (element=w242:sgl)
              n100 = Decrement(x=w246) -> (x-1=w244:i32)
              n101 = call <vilib>:"Derivative x(t) PtByPt.vi"("dt"=10, "x"=w242) -> ()  [unwired: 2 in, 2 out]
              n102 = Decrement(x=w244) -> (x-1=w245:i32)
              n103 = feedback #1() -> (w263:dbl[])
              n104 = Insert Into Array(array=w263, index=w247, new element=w264) -> (w238:dbl[])
              n105 = Multiply(x=w238, y="amplif") -> (x*y=w236:dbl[])
              n106 = feedback-in #1(w238) -> ()
              n107 = feedback #2() -> (w259:dbl[])
              n108 = Insert Into Array(array=w259, index=w247, new element=w260) -> (w240:dbl[])
              n109 = feedback-in #2(w240) -> ()
              n110 = feedback #3() -> (w258:dbl[])
              n111 = Insert Into Array(array=w258, index=w247, new element=w242) -> (w239:dbl[])
              n112 = feedback-in #3(w239) -> ()
              n113 = Array Subset(array=w266, index=0, length=w247) -> (w241:dbl[])
              "Bias Sweep" <- w241
              n114 = Greater Or Equal?(x=w247, y=w245) -> (x >= y?=w249:bool)
              n115 = Subtract(x=w240, y=w239) -> (x-y=w235:dbl[])
              n116 = Bundle(w241, w238) -> (→"IV":cluster{dbl[], dbl[]})  [unwired: 1 in]
              n117 = Bundle(w241, w240) -> (→"dI/dV":cluster{dbl[], dbl[]})  [unwired: 1 in]
              n118 = Bundle(w241, w239) -> (→"d2I/dV2":cluster{dbl[], dbl[]})  [unwired: 1 in]
              n119 = Bundle(w235, w236) -> (→"RTD-IV":cluster{dbl[], dbl[]})  [unwired: 1 in]
              n120 = call <vilib>:"Linear Fit.vi"("Y"=w236, "X"=w235) -> ("slope"=w233:dbl, "intercept"=→"intercept":dbl)  [unwired: 9 in, 3 out]
              n121 = Or(x="Stop Sweep", y=w249) -> (x .or. y?=w248:bool)
              n122 = Reciprocal(x=w233) -> (1/x=w232:dbl)
              "Resistance" <- w232
              "Numeric" <- w247
            }
            n123 = call <vilib>:"DAQmx Clear Task.vi"("task in"=w220, "error in"=w217) -> ("error out"=w216:errorcluster)  [unwired: 13 in]
            n124 = call <vilib>:"DAQmx Clear Task.vi"("task in"=w228, "error in"=w216) -> ("error out"=w215:errorcluster)  [unwired: 13 in]
            n125 = Get Date/Time In Seconds() -> (seconds since 1Jan1904=w167:timestamp)
            n126 = Format Date/Time String(time format string (%c)="%X", seconds (now)=w167) -> (date/time string=w166:string)  [unwired: 1 in]
            "date/time string" <- w166
            n127 = Build Array (concatenate)(w173, w172) -> (w171:dbl[])
            "Array" <- w171
            "Bias Sweep 2" <- w171
            n128 = Build Array (concatenate)(w170, w166) -> (w169:string[])
            n129 = call <vilib>:"General Error Handler.vi"("type of dialog (OK msg:1)"=w219, "error in (no error)"=w215) -> ()  [unwired: 9 in, 5 out]
            n130 = local write "Sweep Bias"(FALSE) -> ()
            "Save Indicator" <- FALSE
          }
          frame 3 {
            w317 = T2 3 items=["no dialog", "OK message", "continue or stop message", "OK message + warnings", "continue/stop + warnings"] ("type of dialog (OK msg:1)")
            w322 = 12522 items=["Finite Samples"=10178, "Continuous Samples"=10123, "Hardware Timed Single Point"=12522] ("sample mode")
            n131 = call-poly <vilib>:"DAQmx Create Virtual Channel.vi"("maximum value"=10.0 ("maximum value 2"), "minimum value"=-10.0 ("minimum value 2"), "physical channels"=tag "Dev1/ao0" ("physical channels 2")) -> ("task out"=w325:refnum<k21>, "error out"=w324:errorcluster)  [unwired: 11 in]
            n132 = call-poly <vilib>:"DAQmx Timing.vi"("task/channels in"=w325, "sample mode"=w322, "rate"=10000, "error in"=w324) -> ("task out"=w321:refnum<k21>, "error out"=w320:errorcluster)  [unwired: 10 in]
            n133 = call <vilib>:"DAQmx Start Task.vi"("task/channels in"=w321, "error in"=w320) -> ("task out"=w319:refnum<k21>, "error out"=w318:errorcluster)  [unwired: 12 in]
            n134 = Add(x=w306, y="Bias Offset Correct") -> (x+y=w307:dbl)
            n135 = call-poly <vilib>:"DAQmx Write.vi"("task/channels in"=w319, "data"=w307, "timeout"=10.0 ("Wirite Timeout"), "error in"=w318) -> ("task out"=w315:refnum<k21>, "error out"=w314:errorcluster)  [unwired: 9 in, 1 out]
            n136 = call <vilib>:"DAQmx Clear Task.vi"("task in"=w315, "error in"=w314) -> ("error out"=w316:errorcluster)  [unwired: 13 in]
            n137 = call <vilib>:"General Error Handler.vi"("type of dialog (OK msg:1)"=w317, "error in (no error)"=w316) -> ()  [unwired: 9 in, 5 out]
          }
          frame 4 {
            n138 = Array Size(array=w332) -> (size(s)=w331:i32)
            "size(s)" <- w331
            n139 = Delete From Array(array=w358, length=2, index (row)=0) -> (array with subset deleted=w355:dbl[][])  [unwired: 1 in, 1 out]
            n140 = Transpose 2D Array(2D array=w355) -> (transposed array=w354:dbl[][])
            n141 = Number To Decimal String(number=w331) -> (decimal integer string=w330:string)  [unwired: 1 in]
            n142 = Build Array (concatenate)(w356, w354) -> (w336:dbl[][])
            n143 = Increment(x="Filenumber") -> (x+1=w381:i32)
            n144 = Format Into String(format string="%03d.txt", initial string="DATA Filename", "Filenumber") -> (resulting string=w369:string)  [unwired: 1 in, 1 out]
            n145 = Transpose 2D Array(2D array=w336) -> (transposed array=w335:dbl[][])
            n146 = Format Into String(format string="%03d.dat", initial string="DATA Filename", "Filenumber") -> (resulting string=w383:string)  [unwired: 1 in, 1 out]
            n147 = Format Into String(format string="%03d.acq", initial string="DATA Filename", "Filenumber") -> (resulting string=w376:string)  [unwired: 1 in, 1 out]
            n148 = Build Path(base path="Data Directory", name or relative path=w369) -> (appended path=w367:path)
            n149 = Build Path(base path="Data Directory", name or relative path=w383) -> (appended path=w380:path)
            n150 = local write "Filenumber"(w381) -> ()
            n151 = Build Path(base path="Data Directory", name or relative path=w376) -> (appended path=w374:path)
            n152 = Concatenate Strings(w330, "\r", "Comment") -> (w352:string)
            n153 = Open/Create/Replace File(file path (use dialog)=w367, operation (0:open)=T1."create") -> (refnum out=w362:refnum<file>)  [unwired: 4 in, 2 out]
            n154 = Open/Create/Replace File(file path (use dialog)=w380, operation (0:open)=T1."create") -> ()  [unwired: 4 in, 3 out]
            n155 = Open/Create/Replace File(file path (use dialog)=w374, operation (0:open)=T1."create") -> (refnum out=w373:refnum<file>)  [unwired: 4 in, 2 out]
            n156 = Write to Text File(file (use dialog)=w362, text=w352) -> (refnum out=w361:refnum<file>)  [unwired: 2 in, 2 out]
            n157 = call-poly <vilib>:"Write To Spreadsheet File.vi"("delimiter (\\t)"=",", "format (%.3f)"="%e", "2D data"=w335, "file path (dialog if empty)"=w380) -> ()  [unwired: 4 in, 1 out]
            n158 = Close File(refnum=w361) -> ()  [unwired: 1 in, 2 out]
            n159 = Array Size(array=w335) -> ()  [unwired: 1 out]
            n160 = Index Array(array=w335, index (col)=0) -> (element=w344:dbl[])  [unwired: 1 in]
            n161 = Index Array(array=w335, index (col)=1) -> (element=w343:dbl[])  [unwired: 1 in]
            n162 = Index Array(array=w335, index (col)=2) -> (element=w342:dbl[])  [unwired: 1 in]
            n163 = Index Array(array=w335, index (col)=5) -> (element=w339:dbl[])  [unwired: 1 in]
            n164 = Index Array(array=w335, index (col)=3) -> (element=w341:dbl[])  [unwired: 1 in]
            n165 = Index Array(array=w335, index (col)=4) -> (element=w340:dbl[])  [unwired: 1 in]
            n166 = Index Array(array=w335, index (col)=6) -> (element=w338:dbl[])  [unwired: 1 in]
            n167 = Bundle(w344, w343, w342, w341, w340, w339, w338) -> ()  [unwired: 1 in, 1 out]
            n168 = Write to Binary File(file (use dialog)=w373, data=w335, 5:TRUE ("prepend array or string size? (T)")) -> (refnum out=w371:refnum<file>)  [unwired: 3 in, 2 out]
            n169 = local write "Save Indicator"(TRUE) -> ()
            n170 = local write "Save IV"(FALSE) -> ()
            n171 = Close File(refnum=w371) -> ()  [unwired: 1 in, 2 out]
          }
          frame 5 {
            n172 = property on="DATA Filename" class="Str"() -> ("Value"=w399:string)  [unwired: 2 in, 2 out]
            n173 = Number To Engineering String(2:i16 8 ("width (-)"), 4:w386) -> (0:w385:string[])  [unwired: 2 in]
            n174 = Concatenate Strings(w399, "_Decay.txt") -> (w403:string)
            n175 = Concatenate Strings(w399, "_Decay.acq") -> (w397:string)
            n176 = property on="Data Directory" class="Path"() -> ("Value"=w396:path)  [unwired: 2 in, 2 out]
            n177 = Build Path(base path=w396, name or relative path=w397) -> (appended path=w395:path)
            n178 = Build Path(base path=w396, name or relative path=w403) -> (appended path=w402:path)
            n179 = Open/Create/Replace File(file path (use dialog)=w395, operation (0:open)=T1."create") -> (refnum out=w401:refnum<file>)  [unwired: 4 in, 2 out]
            n180 = Build Array(w387, w385) -> (w392:string[][])
            n181 = Transpose 2D Array(2D array=w392) -> (transposed array=w391:string[][])
            n182 = Write to Binary File(file (use dialog)=w401, data=w391, 5:FALSE ("prepend array or string size? (T)")) -> (refnum out=w400:refnum<file>)  [unwired: 3 in, 2 out]
            n183 = call-poly <vilib>:"Write To Spreadsheet File.vi"("format (%s)"="%e", "2D data"=w391, "file path (dialog if empty)"=w402) -> ()  [unwired: 5 in, 1 out]
            n184 = Close File(refnum=w400) -> ()  [unwired: 1 in, 2 out]
          }
          frame 6 {
            (unwired) 100000
            w411 = 0.0
            w433 = 10123 items=["Finite Samples"=10178, "Continuous Samples"=10123] ("sample mode")
            w437 = T2 3 items=["no dialog", "OK message", "continue or stop message", "OK message + warnings", "continue/stop + warnings"] ("type of dialog (OK msg:1)")
            w441 = 10123 items=["Finite Samples"=10178, "Continuous Samples"=10123, "Hardware Timed Single Point"=12522] ("sample mode")
            n185 = call-poly <vilib>:"DAQmx Create Virtual Channel.vi"("maximum value"=10.0 ("maximum value 2"), "minimum value"=-10.0 ("minimum value 2"), "physical channels"=tag "Dev1/ao1" ("physical channels 2")) -> ("task out"=w443:refnum<k21>, "error out"=w442:errorcluster)  [unwired: 11 in]
            n186 = call-poly <vilib>:"DAQmx Create Virtual Channel.vi"("maximum value"=10.0 ("Maximum Value 2"), "minimum value"=-10.0 ("Minimum Value 2"), "physical channels"=tag "Dev1/ai0" ("Physical Channel 2")) -> ("task out"=w431:refnum<k21>, "error out"=w432:errorcluster)  [unwired: 11 in]
            n187 = call-poly <vilib>:"DAQmx Timing.vi"("task/channels in"=w431, "sample mode"=w433, "samples per channel"=2, "rate"=5000.0 ("Rate 2"), "error in"=w432) -> ("task out"=w427:refnum<k21>, "error out"=w426:errorcluster)  [unwired: 9 in]
            n188 = call-poly <vilib>:"DAQmx Timing.vi"("task/channels in"=w443, "sample mode"=w441, "rate"=5000, "error in"=w442) -> ("task out"=w440:refnum<k21>, "error out"=w439:errorcluster)  [unwired: 10 in]
            n189 = property class="DAQmx Timing" props=["Sample Clock:Rate"](reference=w427, error in=w426) -> (reference out=w425:refnum<k21>, error out=w424:errorcluster)  [unwired: 1 out]
            n190 = call <vilib>:"DAQmx Start Task.vi"("task/channels in"=w440, "error in"=w439) -> ("task out"=w438:refnum<k21>, "error out"=w420:errorcluster)  [unwired: 12 in]
            n191 = call "Get Terminal Name with Device Prefix.vi"("error in (no error)"=w424, "Local Terminal Name"="ai/StartTrigger" ("terminal"), "task/channels in"=w425) -> ("error out"=w408:errorcluster, "task out"=w409:refnum<k21>)  [unwired: 6 in, 1 out]
            n192 = property on="Waveform Chart" class="WFChart (strict)"("Visible"=TRUE) -> ()  [unwired: 2 in, 2 out]
            n193 = call <vilib>:"DAQmx Start Task.vi"("task/channels in"=w409, "error in"=w408) -> ("task out"=w418:refnum<k21>, "error out"=w422:errorcluster)  [unwired: 12 in]
            n194 = Initialize Array(w411, w411) -> ()  [unwired: 1 out]
            n195 = while {
              tunnel: w438 -> [w469]
              tunnel: w422 -> [w468]
              tunnel: w420 -> [w467]
              tunnel: ["Analog Ouyput 1"] -> w419
              tunnel: w418 -> [w466]
              tunnel: [w465] -> w417
              tunnel: [w464] -> w416
              tunnel: [w463] -> w414
              tunnel: [w457] -> w412
              stop <- w454 stop-if-true
              n196 = call-poly <vilib>:"DAQmx Read.vi"("task/channels in"=w466, "error in"=w468) -> ("task out"=w457:refnum<k21>, "data"=w452:dbl, "error out"=w463:errorcluster)  [unwired: 11 in]
              "Waveform Chart" <- w452
              n197 = call-poly <vilib>:"DAQmx Write.vi"("task/channels in"=w469, "data"="Analog Ouyput 1", "timeout"=0.1 ("Wirite Timeout"), "error in"=w467) -> ("task out"=w465:refnum<k21>, "error out"=w464:errorcluster)  [unwired: 9 in, 1 out]
              n198 = local read "Manual Z"() -> (w451:bool)
              n199 = local read "Sweep Bias"() -> (w455:bool)
              n200 = local read "Save IV"() -> (w453:bool)
              n201 = Build Array("Analog Ouyput 1") -> (w461:dbl[])
              n202 = Build Array(w452) -> (w460:dbl[])
              n203 = Build Array(w460, w461) -> (w459:dbl[][])
              n204 = Not(x=w451) -> (.not. x?=w456:bool)
              n205 = Transpose 2D Array(2D array=w459) -> ()  [unwired: 1 out]
              n206 = Compound Arithmetic op=OR(w453, w455, w456) -> (w454:bool)
            }
            n207 = call <vilib>:"DAQmx Clear Task.vi"("task in"=w417, "error in"=w416) -> ("error out"=w415:errorcluster)  [unwired: 13 in]
            n208 = call <vilib>:"DAQmx Clear Task.vi"("task in"=w412, "error in"=w414) -> ("error out"=w413:errorcluster)  [unwired: 13 in]
            n209 = Merge Errors(w413, w415) -> (w421:errorcluster)
            n210 = call <vilib>:"General Error Handler.vi"("type of dialog (OK msg:1)"=w437, "error in (no error)"=w421) -> ()  [unwired: 9 in, 5 out]
          }
          frame 7 {
            w473 = 0.0
            w494 = T2 3 items=["no dialog", "OK message", "continue or stop message", "OK message + warnings", "continue/stop + warnings"] ("type of dialog (OK msg:1)")
            w509 = 10123 items=["Finite Samples"=10178, "Continuous Samples"=10123] ("sample mode")
            w503 = 10123 items=["Finite Samples"=10178, "Continuous Samples"=10123] ("sample mode")
            n211 = call-poly <vilib>:"DAQmx Create Virtual Channel.vi"("maximum value"=10.0 ("maximum value 2"), "minimum value"=-10.0 ("minimum value 2"), "physical channels"=tag "Dev1/ao1" ("physical channels 2")) -> ("task out"=w510:refnum<k21>, "error out"=w511:errorcluster)  [unwired: 11 in]
            n212 = call-poly <vilib>:"DAQmx Create Virtual Channel.vi"("maximum value"=10.0 ("Maximum Value 2"), "minimum value"=-10.0 ("Minimum Value 2"), "physical channels"=tag "Dev1/ai0" ("Physical Channel 2")) -> ("task out"=w505:refnum<k21>, "error out"=w504:errorcluster)  [unwired: 11 in]
            n213 = call-poly <vilib>:"DAQmx Timing.vi"("task/channels in"=w510, "sample mode"=w509, "rate"=10000.0 ("rate 2"), "error in"=w511) -> ("task out"=w518:refnum<k21>, "error out"=w519:errorcluster)  [unwired: 10 in]
            n214 = call-poly <vilib>:"DAQmx Timing.vi"("task/channels in"=w505, "sample mode"=w503, "rate"=10000.0 ("Rate 2"), "error in"=w504) -> ("task out"=w521:refnum<k21>, "error out"=w522:errorcluster)  [unwired: 10 in]
            n215 = property class="DAQmx Timing" props=["Sample Clock:Rate"](reference=w518, error in=w519) -> (reference out=w517:refnum<k21>, error out=w520:errorcluster)  [unwired: 1 out]
            n216 = property class="DAQmx Timing" props=["Sample Clock:Rate"](reference=w521, error in=w522) -> (reference out=w523:refnum<k21>, error out=w524:errorcluster)  [unwired: 1 out]
            n217 = call "Get Terminal Name with Device Prefix.vi"("error in (no error)"=w524, "Local Terminal Name"="ai/StartTrigger" ("terminal"), "task/channels in"=w523) -> ("error out"=w492:errorcluster, "Terminal Name with Device Prefix"=w516:tag, "task out"=w490:refnum<k21>)  [unwired: 6 in]
            n218 = call-poly <vilib>:"DAQmx Trigger.vi"("task/channels in"=w517, "source"=w516, "error in"=w520) -> ("task out"=w485:refnum<k21>, "error out"=w482:errorcluster)  [unwired: 11 in]
            n219 = Initialize Array(0.0, "Step Length") -> (w488:dbl[])
            n220 = call <vilib>:"DAQmx Start Task.vi"("task/channels in"=w490, "error in"=w492) -> ("task out"=w489:refnum<k21>, "error out"=w491:errorcluster)  [unwired: 12 in]
            n221 = call <vilib>:"DAQmx Start Task.vi"("task/channels in"=w485, "error in"=w482) -> ("task out"=w484:refnum<k21>, "error out"=w483:errorcluster)  [unwired: 12 in]
            n222 = Initialize Array(w473, w473) -> (w472:dbl[])
            n223 = while {
              tunnel: w489 -> [w545]
              tunnel: w491 -> [w544]
              tunnel: w484 -> [w543]
              tunnel: w483 -> [w542]
              tunnel: [w541] -> w500
              tunnel: [w540] -> w499
              tunnel: [w539] -> w497
              tunnel: [w538] -> w495
              shift-right: [w536] -> _
              shift-left: w488 -> [w537]
              tunnel: w480 -> [w534]
              shift-right: [w533] -> _
              shift-left: 1 -> [w532]
              shift-right: [w531] -> w476
              shift-left: w481 -> [w535]
              shift-right: [w529] -> w475
              shift-left: w472 -> [w530]
              shift-right: [w527] -> w474
              shift-left: w472 -> [w528]
              tunnel: [w525] -> w471
              stop <- w525 stop-if-true
              n224 = stacked-sequence {
                seq-local: [w547 _] -> [_ w587]
                tunnel: w545 -> [w578 _]
                tunnel: w544 -> [w577 _]
                tunnel: w543 -> [_ w595]
                tunnel: w542 -> [_ w594]
                tunnel: [w575 _] -> w541
                tunnel: [w576 _] -> w540
                tunnel: [_ w592] -> w539
                tunnel: [_ w593] -> w538
                tunnel: w537 -> [w572 w579]
                tunnel: [w555 _] -> w536
                tunnel: [w548 _] -> w525
                tunnel: w535 -> [_ w591]
                tunnel: w534 -> [_ w590]
                tunnel: [_ w589] -> w533
                tunnel: w532 -> [w564 w588]
                tunnel: "Ramp Rate" -> [_ w586]
                tunnel: [_ w584] -> _
                tunnel: [_ w584] -> w531
                tunnel: w530 -> [_ w583]
                tunnel: [_ w582] -> w529
                tunnel: w528 -> [_ w581]
                tunnel: [_ w580] -> w527
                frame #0 {
                  n225 = call-poly <vilib>:"DAQmx Read.vi"("task/channels in"=w578, "error in"=w577) -> ("task out"=w575:refnum<k21>, "data"=w546:dbl, "error out"=w576:errorcluster)  [unwired: 11 in]
                  n226 = Absolute Value(x=w546) -> (abs(x)=w547:dbl)
                  n227 = Insert Into Array(array=w572, index=0, new element=w547) -> (w573:dbl[])
                  n228 = local write "Waveform Chart"(w547) -> ()
                  n229 = Delete From Array(array=w573, length=1) -> (array with subset deleted=w555:dbl[])  [unwired: 1 in, 1 out]
                  n230 = Array Size(array=w555) -> (size(s)=w565:i32)
                  n231 = Decrement(x=w565) -> (x-1=w556:i32)
                  n232 = Index Array(array=w555, index=w556) -> (element=w558:dbl)
                  "element" <- w558
                  n233 = Index Array(array=w555, index=0) -> (element=w560:dbl)
                  n234 = Less?(x=w555, y="Step Max") -> (x < y?=w570:bool[])
                  n235 = Greater?(x=w555, y="Step Min") -> (0:w569:bool[])
                  n236 = Greater?(x="Step Min", y=w558) -> ()  [unwired: 1 out]
                  n237 = And Array Elements(Boolean array=w570) -> (logical AND=w554:bool)
                  n238 = And Array Elements(Boolean array=w569) -> (logical AND=w553:bool)
                  n239 = Less?(x="Step Max", y=w560) -> ()  [unwired: 1 out]
                  n240 = local read "Tapping"() -> (w550:bool)
                  n241 = And(x=w554, y=w553) -> (x .and. y?=w568:bool)
                  n242 = Equal?(x=w564, y=1) -> (x = y?=w562:bool)
                  n243 = Equal?(x=w564, y=2) -> (x = y?=w561:bool)
                  n244 = Or(x=w562, y=w561) -> (x .or. y?=w552:bool)
                  n245 = Not(x=w550) -> (.not. x?=w549:bool)
                  n246 = Compound Arithmetic op=AND(w568, w552) -> (w551:bool)
                  "Tapping Stop" <- w551
                  n247 = Or(x=w551, y=w549) -> (x .or. y?=w548:bool)
                }
                frame #1 {
                  n248 = case shown="1, Default" w588 {
                    tunnel: [w603 w626 w647 w673] -> w584
                    tunnel: w591 -> [w616 w628 w658 w670]
                    tunnel: [w611 w627 w652 w669] -> w589
                    tunnel: w587 -> [w602 _ w657 _]
                    tunnel: w586 -> [w617 w631 w659 w668]
                    tunnel: w583 -> [w607 w625 w646 _]
                    tunnel: [w609 w625 w646 w666] -> w582
                    tunnel: w581 -> [w601 w624 w645 _]
                    tunnel: [w608 w624 w645 w666] -> w580
                    tunnel: w579 -> [w600 _ _ _]
                    frame 1, Default {
                      w605 = -10
                      # "Breaking the contact"
                      n249 = Divide(x=w617, y=15.13) -> (x/y=w621:dbl)
                      n250 = Array Subset(array=w600, index=0, length=10) -> (w597:dbl[])
                      n251 = Divide(x=20, y=32768) -> (x/y=w618:dbl)
                      n252 = call-poly <vilib>:"Mean.vi"("X"=w597) -> ("mean"=w596:dbl)  [unwired: 1 out]
                      "mean" <- w596
                      n253 = Multiply(x=w618, y=w621) -> (x*y=w623:dbl)
                      n254 = Subtract(x=w616, y=w623) -> (x-y=w604:dbl)
                      n255 = Less?(x=w596, y="Min Current") -> (x < y?=w614:bool)
                      n256 = Select(t=2, s=w614, f=1) -> (s? t:f=w611:i32)
                      n257 = Build Array (concatenate)(w604, w607) -> (w609:dbl[])
                      n258 = Build Array (concatenate)(w602, w601) -> (w608:dbl[])
                      n259 = Less?(x=w604, y=w605) -> (x < y?=w606:bool)
                      n260 = local write "Contact Cycles"(0) -> ()
                      n261 = Select(t=w605, s=w606, f=w604) -> (s? t:f=w603:dbl)
                    }
                    frame 2 {
                      w643 = 10
                      # "Break contact cycles after current = 0"
                      n262 = Divide(x=w631, y=15.13) -> (x/y=w639:dbl)
                      n263 = local read "Contact Cycles"() -> (w630:i32)
                      n264 = Divide(x=20, y=32768) -> (x/y=w632:dbl)
                      n265 = Multiply(x=w632, y=w639) -> (x*y=w641:dbl)
                      n266 = Subtract(x=w628, y=w641) -> (x-y=w633:dbl)
                      n267 = Increment(x=w630) -> (x+1=w629:i32)
                      n268 = Less?(x=w633, y=w643) -> (x < y?=w642:bool)
                      n269 = Select(t=w633, s=w642, f=w643) -> (s? t:f=w626:dbl)
                      n270 = Less Or Equal?(x="Break Contact", y=w629) -> (x <= y?=w636:bool)
                      n271 = local write "Contact Cycles"(w629) -> ()
                      n272 = Select(t=3, s=w636, f=2) -> (s? t:f=w627:i32)
                    }
                    frame 3 {
                      w650 = 10
                      # "Making contact"
                      n273 = Divide(x=w659, y=15.13) -> (x/y=w663:dbl)
                      n274 = Divide(x=20, y=32768) -> (x/y=w660:dbl)
                      n275 = Multiply(x=w660, y=w663) -> (x*y=w665:dbl)
                      n276 = Add(x=w658, y=w665) -> (x+y=w648:dbl)
                      n277 = Greater?(x=w657, y="Max Current") -> (0:w655:bool)
                      n278 = Select(t=4, s=w655, f=3) -> (s? t:f=w652:i32)
                      n279 = local write "Contact Cycles"(0) -> ()
                      n280 = Less?(x=w648, y=w650) -> (x < y?=w649:bool)
                      n281 = Select(t=w648, s=w649, f=w650) -> (s? t:f=w647:dbl)
                    }
                    frame 4 {
                      w667 = 0.0
                      w685 = 10
                      # "Make contact cycles after current saturation"
                      n282 = Divide(x=w668, y=15.13) -> (x/y=w681:dbl)
                      n283 = local read "Contact Cycles"() -> (w675:i32)
                      n284 = Divide(x=20, y=32768) -> (x/y=w671:dbl)
                      n285 = Multiply(x=w671, y=w681) -> (x*y=w683:dbl)
                      n286 = Add(x=w670, y=w683) -> (x+y=w672:dbl)
                      n287 = Increment(x=w675) -> (x+1=w674:i32)
                      n288 = Less?(x=w672, y=w685) -> (x < y?=w684:bool)
                      n289 = Select(t=w672, s=w684, f=w685) -> (s? t:f=w673:dbl)
                      n290 = Less Or Equal?(x="Make Contact", y=w674) -> (x <= y?=w678:bool)
                      n291 = local write "Contact Cycles"(w674) -> ()
                      n292 = Initialize Array(w667, w667) -> (w666:dbl[])
                      n293 = Select(t=1, s=w678, f=4) -> (s? t:f=w669:i32)
                    }
                  }
                  n294 = local write "Analog Ouyput 1"(w584) -> ()
                  n295 = Build Array(w590, w584) -> ()  [unwired: 1 out]
                  n296 = call-poly <vilib>:"DAQmx Write.vi"("task/channels in"=w595, "auto start"=TRUE, "data"=w584, "error in"=w594) -> ("task out"=w593:refnum<k21>, "error out"=w592:errorcluster)  [unwired: 9 in, 1 out]
                }
              }
              "Case" <- w533
            }
            n297 = call <vilib>:"DAQmx Clear Task.vi"("task in"=w495, "error in"=w497) -> ("error out"=w496:errorcluster)  [unwired: 13 in]
            n298 = Not(x=w471) -> (.not. x?=w470:bool)
            n299 = call <vilib>:"DAQmx Clear Task.vi"("task in"=w500, "error in"=w499) -> ("error out"=w498:errorcluster)  [unwired: 13 in]
            n300 = local write "Tapping"(w470) -> ()
            n301 = Merge Errors(w498, w496) -> (w493:errorcluster)
            n302 = call <vilib>:"General Error Handler.vi"("type of dialog (OK msg:1)"=w494, "error in (no error)"=w493) -> ()  [unwired: 9 in, 5 out]
          }
          frame 8 {
            w692 = 0.0
            w706 = T2 3 items=["no dialog", "OK message", "continue or stop message", "OK message + warnings", "continue/stop + warnings"] ("type of dialog (OK msg:1)")
            w719 = 10123 items=["Finite Samples"=10178, "Continuous Samples"=10123] ("sample mode")
            w713 = 10123 items=["Finite Samples"=10178, "Continuous Samples"=10123] ("sample mode")
            n303 = call-poly <vilib>:"DAQmx Create Virtual Channel.vi"("maximum value"=10.0 ("maximum value 2"), "minimum value"=-10.0 ("minimum value 2"), "physical channels"=tag "Dev1/ao0:1" ("physical channels 2")) -> ("task out"=w720:refnum<k21>, "error out"=w721:errorcluster)  [unwired: 11 in]
            n304 = call-poly <vilib>:"DAQmx Create Virtual Channel.vi"("maximum value"=10.0 ("Maximum Value 2"), "minimum value"=-10.0 ("Minimum Value 2"), "physical channels"=tag "Dev1/ai0" ("Physical Channel 2")) -> ("task out"=w715:refnum<k21>, "error out"=w714:errorcluster)  [unwired: 11 in]
            n305 = call-poly <vilib>:"DAQmx Timing.vi"("task/channels in"=w720, "sample mode"=w719, "rate"=10000.0 ("rate 2"), "error in"=w721) -> ("task out"=w728:refnum<k21>, "error out"=w729:errorcluster)  [unwired: 10 in]
            n306 = call-poly <vilib>:"DAQmx Timing.vi"("task/channels in"=w715, "sample mode"=w713, "rate"=10000.0 ("Rate 2"), "error in"=w714) -> ("task out"=w731:refnum<k21>, "error out"=w732:errorcluster)  [unwired: 10 in]
            n307 = property class="DAQmx Timing" props=["Sample Clock:Rate"](reference=w728, error in=w729) -> (reference out=w727:refnum<k21>, error out=w730:errorcluster)  [unwired: 1 out]
            n308 = property class="DAQmx Timing" props=["Sample Clock:Rate"](reference=w731, error in=w732) -> (reference out=w733:refnum<k21>, error out=w734:errorcluster)  [unwired: 1 out]
            n309 = call "Get Terminal Name with Device Prefix.vi"("error in (no error)"=w734, "Local Terminal Name"="ai/StartTrigger" ("terminal"), "task/channels in"=w733) -> ("error out"=w704:errorcluster, "Terminal Name with Device Prefix"=w726:tag, "task out"=w702:refnum<k21>)  [unwired: 6 in]
            n310 = call-poly <vilib>:"DAQmx Trigger.vi"("task/channels in"=w727, "source"=w726, "error in"=w730) -> ("task out"=w700:refnum<k21>, "error out"=w697:errorcluster)  [unwired: 11 in]
            n311 = call <vilib>:"DAQmx Start Task.vi"("task/channels in"=w702, "error in"=w704) -> ("task out"=w701:refnum<k21>, "error out"=w703:errorcluster)  [unwired: 12 in]
            n312 = call <vilib>:"DAQmx Start Task.vi"("task/channels in"=w700, "error in"=w697) -> ("task out"=w699:refnum<k21>, "error out"=w698:errorcluster)  [unwired: 12 in]
            n313 = Initialize Array(w692, w692) -> ()  [unwired: 1 out]
            n314 = while {
              tunnel: w701 -> [w769]
              tunnel: w703 -> [w768]
              tunnel: w699 -> [w758]
              tunnel: w698 -> [w757]
              tunnel: [w767] -> w710
              tunnel: [w766] -> w709
              shift-right: [w743] -> w693
              shift-left: w696 -> [w748]
              tunnel: [w756] -> w691
              tunnel: [w755] -> w690
              tunnel: w687 -> [w739]
              i -> [w754]
              stop <- w744 stop-if-true
              w752 = 5e-05
              n315 = Absolute Value(x="Setpoint") -> (abs(x)=w735:dbl)
              n316 = call-poly <vilib>:"DAQmx Read.vi"("task/channels in"=w769, "error in"=w768) -> ("task out"=w767:refnum<k21>, "data"=w738:dbl, "error out"=w766:errorcluster)  [unwired: 11 in]
              n317 = Absolute Value(x=w738) -> (abs(x)=w737:dbl)
              n318 = local read "Bias Offset Correct"() -> (w740:dbl)
              n319 = Bundle("Proportional Gain"="Proportional Gain", "Integral Gain"="Integral Gain", "Differential Gain"="Differential Gain") -> (w759:T3)  [unwired: 1 in]
              n320 = local write "Waveform Chart"(w738) -> ()
              n321 = Bundle(10, -10) -> (w763:cluster{i32, i32})  [unwired: 1 in]
              n322 = call-poly "PID.vi"("output range"=w763, "dt (s)"=w752, "PID gains"=w759, "process variable"=w737, "setpoint"=w735) -> ("output"=w751:dbl)  [unwired: 5 in, 1 out]
              n323 = Add(x=w739, y=w740) -> (x+y=w741:dbl)
              n324 = Less?(x=w754, y=1000) -> (x < y?=w749:bool)
              n325 = call-poly "PID Output Rate Limiter.vi"("reinitialize? (F)"=w749, "dt (s)"=w752, "output rate (EGU/min)"="Piezo Delta rate", "initial output"=w748, "input (controller output)"=w751) -> ("output"=w743:dbl)  [unwired: 3 in, 1 out]
              n326 = local write "Analog Ouyput 1"(w743) -> ()
              n327 = Build Array(w741, w743) -> (w742:dbl[])
              n328 = local read "Sweep Bias"() -> (w747:bool)
              n329 = local read "PID"() -> (w745:bool)
              n330 = call-poly <vilib>:"DAQmx Write.vi"("task/channels in"=w758, "data"=w742, "error in"=w757) -> ("task out"=w756:refnum<k21>, "error out"=w755:errorcluster)  [unwired: 10 in, 1 out]
              n331 = Not(x=w745) -> (.not. x?=w746:bool)
              n332 = Compound Arithmetic op=OR(w747, w746) -> (w744:bool)
            }
            n333 = call <vilib>:"DAQmx Clear Task.vi"("task in"=w691, "error in"=w690) -> ("error out"=w707:errorcluster)  [unwired: 13 in]
            n334 = call <vilib>:"DAQmx Clear Task.vi"("task in"=w710, "error in"=w709) -> ("error out"=w708:errorcluster)  [unwired: 13 in]
            n335 = Merge Errors(w708, w707) -> (w705:errorcluster)
            n336 = call <vilib>:"General Error Handler.vi"("type of dialog (OK msg:1)"=w706, "error in (no error)"=w705) -> ()  [unwired: 9 in, 5 out]
          }
        }
      }
    }
  }
